vi "FeedbackDecode_MLComCtrl.vi"(6 "CognitiveLoadIn":T1, 8 "DecodeClustIn":T4={"TrainParams"={"Lag"=0.0, "KernelWidth"=0.3, "TargRad"=0.15}, "Kinematics"={"Thumb"=0.0, "Index"=0.0, "Middle"=0.0, "Ring"=0.0, "Little"=0.0, "ThumbInt"=0.0, "IndexInt"=0.0, "RingInt"=0.0, "LittleInt"=0.0, "Wrist"=0.0, "WristYaw"=0.0, "WristRoll"=0.0}, "CtrlButtons"={"AcqTraining"=FALSE, "ApplyBaseline"=FALSE, "ApplyTraining"=FALSE, "LoadTrainFile"=FALSE, "CAR"=FALSE, "NIPSpikes"=FALSE, "AcqBaseline"=FALSE, "Stop"=FALSE, "ResetTrial"=FALSE, "CalDEKA"=FALSE, "HideSphrs"=FALSE, "StartTrials"=FALSE, "AutoPop"=FALSE, "ResetVRE"=FALSE, "StopVRE"=FALSE, "AcqCAR"=FALSE, "ConARD"=FALSE, "DEKARestart"=FALSE, "ConnDEKA"=FALSE}, "CompID"={"LV"={"Name"="PNILABVIEW", "IP"="155.100.90.215"}, "ML"={"Name"="PNIMATLAB", "IP"="155.100.91.231"}}, "KMvntClust"={"KGain"=[[1.0, 1.0, -1.0, 1.0], [1.0, 1.0, -1.0, 1.0], [1.0, 1.0, -1.0, 1.0], [1.0, 1.0, -1.0, 1.0], [1.0, 1.0, -1.0, 1.0], [1.0, 1.0, -1.0, 1.0], [1.0, 1.0, -1.0, 1.0], [1.0, 1.0, -1.0, 1.0], [1.0, 1.0, -1.0, 1.0], [1.0, 1.0, -1.0, 1.0], [1.0, 1.0, -1.0, 1.0], [1.0, 1.0, -1.0, 1.0]], "KMvnts"={"Thumb"=FALSE, "Index"=FALSE, "Middle"=FALSE, "Ring"=FALSE, "Little"=FALSE, "ThumbInt"=FALSE, "IndexInt"=FALSE, "RingInt"=FALSE, "LittleInt"=FALSE, "WristPitch"=FALSE, "WristYaw"=FALSE, "WristRoll"=FALSE}, "KThresh"=[[0.2, 0.2, -1.0, 1.0], [0.2, 0.2, -1.0, 1.0], [0.2, 0.2, -1.0, 1.0], [0.2, 0.2, -1.0, 1.0], [0.2, 0.2, -1.0, 1.0], [0.2, 0.2, -1.0, 1.0], [0.2, 0.2, -1.0, 1.0], [0.2, 0.2, -1.0, 1.0], [0.2, 0.2, -1.0, 1.0], [0.2, 0.2, -1.0, 1.0], [0.2, 0.2, -1.0, 1.0], [0.2, 0.2, -1.0, 1.0]], "CtrlMode"=[], "CtrlSpd"=[]}, "ClearUEA"=FALSE, "Targets"={"Thumb"=0.0, "Index"=0.0, "Middle"=0.0, "Ring"=0.0, "Little"=0.0, "ThumbInt"=0.0, "IndexInt"=0.0, "RingInt"=0.0, "LittleInt"=0.0, "Wrist"=0.0, "WristYaw"=0.0, "WristRoll"=0.0}, "KUEAArray"=[{"Boolean 1"=FALSE, "Boolean 2"=FALSE, "Boolean 3"=FALSE, "Boolean 4"=FALSE, "Boolean 5"=FALSE, "Boolean 6"=FALSE, "Boolean 7"=FALSE, "Boolean 8"=FALSE, "Boolean 9"=FALSE, "Boolean 10"=FALSE, "Boolean 11"=FALSE, "Boolean 12"=FALSE, "Boolean 13"=FALSE, "Boolean 14"=FALSE, "Boolean 15"=FALSE, "Boolean 16"=FALSE, "Boolean 17"=FALSE, "Boolean 18"=FALSE, "Boolean 19"=FALSE, "Boolean 20"=FALSE, "Boolean 21"=FALSE, "Boolean 22"=FALSE, "Boolean 23"=FALSE, "Boolean 24"=FALSE, "Boolean 25"=FALSE, "Boolean 26"=FALSE, "Boolean 27"=FALSE, "Boolean 28"=FALSE, "Boolean 29"=FALSE, "Boolean 30"=FALSE, "Boolean 31"=FALSE, "Boolean 32"=FALSE, "Boolean 33"=FALSE, "Boolean 34"=FALSE, "Boolean 35"=FALSE, "Boolean 36"=FALSE, "Boolean 37"=FALSE, "Boolean 38"=FALSE, "Boolean 39"=FALSE, "Boolean 40"=FALSE, "Boolean 41"=FALSE, "Boolean 42"=FALSE, "Boolean 43"=FALSE, "Boolean 44"=FALSE, "Boolean 45"=FALSE, "Boolean 46"=FALSE, "Boolean 47"=FALSE, "Boolean 48"=FALSE, "Boolean 49"=FALSE, "Boolean 50"=FALSE, "Boolean 51"=FALSE, "Boolean 52"=FALSE, "Boolean 53"=FALSE, "Boolean 54"=FALSE, "Boolean 55"=FALSE, "Boolean 56"=FALSE, "Boolean 57"=FALSE, "Boolean 58"=FALSE, "Boolean 59"=FALSE, "Boolean 60"=FALSE, "Boolean 61"=FALSE, "Boolean 62"=FALSE, "Boolean 63"=FALSE, "Boolean 64"=FALSE, "Boolean 65"=FALSE, "Boolean 66"=FALSE, "Boolean 67"=FALSE, "Boolean 68"=FALSE, "Boolean 69"=FALSE, "Boolean 70"=FALSE, "Boolean 71"=FALSE, "Boolean 72"=FALSE, "Boolean 73"=FALSE, "Boolean 74"=FALSE, "Boolean 75"=FALSE, "Boolean 76"=FALSE, "Boolean 77"=FALSE, "Boolean 78"=FALSE, "Boolean 79"=FALSE, "Boolean 80"=FALSE, "Boolean 81"=FALSE, "Boolean 82"=FALSE, "Boolean 83"=FALSE, "Boolean 84"=FALSE, "Boolean 85"=FALSE, "Boolean 86"=FALSE, "Boolean 87"=FALSE, "Boolean 88"=FALSE, "Boolean 89"=FALSE, "Boolean 90"=FALSE, "Boolean 91"=FALSE, "Boolean 92"=FALSE, "Boolean 93"=FALSE, "Boolean 94"=FALSE, "Boolean 95"=FALSE, "Boolean 96"=FALSE, "Boolean 97"=FALSE, "Boolean 98"=FALSE, "Boolean 99"=FALSE, "Boolean 100"=FALSE}, {"Boolean 1"=FALSE, "Boolean 2"=FALSE, "Boolean 3"=FALSE, "Boolean 4"=FALSE, "Boolean 5"=FALSE, "Boolean 6"=FALSE, "Boolean 7"=FALSE, "Boolean 8"=FALSE, "Boolean 9"=FALSE, "Boolean 10"=FALSE, "Boolean 11"=FALSE, "Boolean 12"=FALSE, "Boolean 13"=FALSE, "Boolean 14"=FALSE, "Boolean 15"=FALSE, "Boolean 16"=FALSE, "Boolean 17"=FALSE, "Boolean 18"=FALSE, "Boolean 19"=FALSE, "Boolean 20"=FALSE, "Boolean 21"=FALSE, "Boolean 22"=FALSE, "Boolean 23"=FALSE, "Boolean 24"=FALSE, "Boolean 25"=FALSE, "Boolean 26"=FALSE, "Boolean 27"=FALSE, "Boolean 28"=FALSE, "Boolean 29"=FALSE, "Boolean 30"=FALSE, "Boolean 31"=FALSE, "Boolean 32"=FALSE, "Boolean 33"=FALSE, "Boolean 34"=FALSE, "Boolean 35"=FALSE, "Boolean 36"=FALSE, "Boolean 37"=FALSE, "Boolean 38"=FALSE, "Boolean 39"=FALSE, "Boolean 40"=FALSE, "Boolean 41"=FALSE, "Boolean 42"=FALSE, "Boolean 43"=FALSE, "Boolean 44"=FALSE, "Boolean 45"=FALSE, "Boolean 46"=FALSE, "Boolean 47"=FALSE, "Boolean 48"=FALSE, "Boolean 49"=FALSE, "Boolean 50"=FALSE, "Boolean 51"=FALSE, "Boolean 52"=FALSE, "Boolean 53"=FALSE, "Boolean 54"=FALSE, "Boolean 55"=FALSE, "Boolean 56"=FALSE, "Boolean 57"=FALSE, "Boolean 58"=FALSE, "Boolean 59"=FALSE, "Boolean 60"=FALSE, "Boolean 61"=FALSE, "Boolean 62"=FALSE, "Boolean 63"=FALSE, "Boolean 64"=FALSE, "Boolean 65"=FALSE, "Boolean 66"=FALSE, "Boolean 67"=FALSE, "Boolean 68"=FALSE, "Boolean 69"=FALSE, "Boolean 70"=FALSE, "Boolean 71"=FALSE, "Boolean 72"=FALSE, "Boolean 73"=FALSE, "Boolean 74"=FALSE, "Boolean 75"=FALSE, "Boolean 76"=FALSE, "Boolean 77"=FALSE, "Boolean 78"=FALSE, "Boolean 79"=FALSE, "Boolean 80"=FALSE, "Boolean 81"=FALSE, "Boolean 82"=FALSE, "Boolean 83"=FALSE, "Boolean 84"=FALSE, "Boolean 85"=FALSE, "Boolean 86"=FALSE, "Boolean 87"=FALSE, "Boolean 88"=FALSE, "Boolean 89"=FALSE, "Boolean 90"=FALSE, "Boolean 91"=FALSE, "Boolean 92"=FALSE, "Boolean 93"=FALSE, "Boolean 94"=FALSE, "Boolean 95"=FALSE, "Boolean 96"=FALSE, "Boolean 97"=FALSE, "Boolean 98"=FALSE, "Boolean 99"=FALSE, "Boolean 100"=FALSE}], "ReTrain"=FALSE, "TargDist"=[0.0, 0.0, 0.0, 0.0, 0.0, 0.0], "State"=enum."Initialize", "KalmanType"=enum."Standard", "EventStr"="", "SelElect"=1.0, "KinSrc"=enum."Training", "HoverElect"=0.0, "RasterWin"=1.0, "WfCnt"=15.0, "ClearWfs"=FALSE, "ApplyThresh"=FALSE, "ThreshVal"=-5.0, "ThreshMode"=enum."RMS Single", "DataFolder"="00000000-000000", "ClearEMG"=FALSE, "KEMGClust"={"Boolean 92"=FALSE, "Boolean 82"=FALSE, "Boolean 72"=FALSE, "Boolean 62"=FALSE, "Boolean 52"=FALSE, "Boolean 42"=FALSE, "Boolean 32"=FALSE, "Boolean 22"=FALSE, "Boolean 12"=FALSE, "Boolean 2"=FALSE, "Boolean 93"=FALSE, "Boolean 83"=FALSE, "Boolean 73"=FALSE, "Boolean 63"=FALSE, "Boolean 53"=FALSE, "Boolean 43"=FALSE, "Boolean 33"=FALSE, "Boolean 23"=FALSE, "Boolean 13"=FALSE, "Boolean 3"=FALSE, "Boolean 94"=FALSE, "Boolean 84"=FALSE, "Boolean 74"=FALSE, "Boolean 64"=FALSE, "Boolean 54"=FALSE, "Boolean 44"=FALSE, "Boolean 34"=FALSE, "Boolean 24"=FALSE, "Boolean 14"=FALSE, "Boolean 4"=FALSE, "Boolean 95"=FALSE, "Boolean 85"=FALSE, "Boolean 75"=FALSE, "Boolean 65"=FALSE, "Boolean 55"=FALSE, "Boolean 45"=FALSE, "Boolean 35"=FALSE, "Boolean 25"=FALSE, "Boolean 15"=FALSE, "Boolean 5"=FALSE, "Boolean 96"=FALSE, "Boolean 86"=FALSE, "Boolean 76"=FALSE, "Boolean 66"=FALSE, "Boolean 56"=FALSE, "Boolean 46"=FALSE, "Boolean 36"=FALSE, "Boolean 26"=FALSE, "Boolean 16"=FALSE, "Boolean 6"=FALSE, "Boolean 97"=FALSE, "Boolean 87"=FALSE, "Boolean 77"=FALSE, "Boolean 67"=FALSE, "Boolean 57"=FALSE, "Boolean 47"=FALSE, "Boolean 37"=FALSE, "Boolean 27"=FALSE, "Boolean 17"=FALSE, "Boolean 7"=FALSE, "Boolean 98"=FALSE, "Boolean 88"=FALSE, "Boolean 78"=FALSE, "Boolean 68"=FALSE, "Boolean 58"=FALSE, "Boolean 48"=FALSE, "Boolean 38"=FALSE, "Boolean 28"=FALSE, "Boolean 18"=FALSE, "Boolean 8"=FALSE, "Boolean 99"=FALSE, "Boolean 89"=FALSE, "Boolean 79"=FALSE, "Boolean 69"=FALSE, "Boolean 59"=FALSE, "Boolean 49"=FALSE, "Boolean 39"=FALSE, "Boolean 29"=FALSE, "Boolean 19"=FALSE, "Boolean 9"=FALSE}, "EvntFlag"=FALSE, "FillUEA"=FALSE, "FillEMG"=FALSE, "FillMvnts"=FALSE, "BadUEAElects"=[], "KEMGExtra"=[], "AllPairs"=FALSE, "AutoThresh"=0.4, "BadEMGChans"=[], "LinkedDOF"="{}", "AutoPopType"=enum."Standard", "CARType"=enum."Standard", "*Map"=enum."pNeural/pEMG", "GainFill"=1.0, "ThreshFill"=1.0, "TestType"=enum."MSMS", "Outcome"=enum."---", "TrialCnt"=[], "ClearTrials"=FALSE, "Log10"=FALSE, "KDFFile"="{}", "LimitExt"=FALSE, "*Prosthesis"=enum."MaleLeft", "StartML"=FALSE, "StartMLAux"=FALSE, "StartRec"=FALSE, "DynaThr"=FALSE, "ModeFill"=enum."Position", "SpdFill"=1.0, "DEKAMode"=enum."Velocity", "FreeParam"=0.4, "GoalNoise"=0.4, "Load NN"=FALSE, "ExportTrain"=FALSE, "NumComp"=enum."2 Computers", "DataDir"="00000000-000000", "BuildDir"="00000000-000000", "LatchingFilter"=FALSE, "Trigger"=FALSE, "StartARD"=FALSE, "StartTaska"=FALSE, "StartTaskaSens"=FALSE} {"SpdFill" min=0.0 max=10.0 step=0.1; "RasterWin" min=1.0 max=30.0 step=1.0; "ThreshFill" min=0.0 max=10.0 step=0.01; "GainFill" min=0.0 max=10.0 step=0.1; "AutoThresh" min=0.0 max=1.0; "Targets"."LittleInt" min=0.0 max=1.0 step=0.01; "Targets"."WristRoll" min=0.0 max=1.0 step=0.01; "Targets"."WristYaw" min=0.0 max=1.0 step=0.01; "Targets"."Wrist" min=0.0 max=1.0 step=0.01; "Targets"."Little" min=0.0 max=1.0 step=0.01; "Targets"."Thumb" min=0.0 max=1.0 step=0.01; "Targets"."RingInt" min=0.0 max=1.0 step=0.01; "Targets"."IndexInt" min=0.0 max=1.0 step=0.01; "Targets"."ThumbInt" min=0.0 max=1.0 step=0.01; "Targets"."Ring" min=0.0 max=1.0 step=0.01; "Targets"."Middle" min=0.0 max=1.0 step=0.01; "Targets"."Index" min=0.0 max=1.0 step=0.01; "KMvntClust"."CtrlSpd" min=0 max=10; "KMvntClust"."KThresh" min=0 max=1; "KMvntClust"."KGain" min=0; "Kinematics"."LittleInt" min=0.0 max=1.0 step=0.01; "Kinematics"."WristRoll" min=0.0 max=1.0 step=0.01; "Kinematics"."WristYaw" min=0.0 max=1.0 step=0.01; "Kinematics"."Wrist" min=0.0 max=1.0 step=0.01; "Kinematics"."Little" min=0.0 max=1.0 step=0.01; "Kinematics"."Thumb" min=0.0 max=1.0 step=0.01; "Kinematics"."RingInt" min=0.0 max=1.0 step=0.01; "Kinematics"."IndexInt" min=0.0 max=1.0 step=0.01; "Kinematics"."ThumbInt" min=0.0 max=1.0 step=0.01; "Kinematics"."Ring" min=0.0 max=1.0 step=0.01; "Kinematics"."Middle" min=0.0 max=1.0 step=0.01; "Kinematics"."Index" min=0.0 max=1.0 step=0.01; "TrainParams"."TargRad" step=0.05 format="%#.2g"; "TrainParams"."KernelWidth" step=0.05 format="%#.2g"}, 9 "EncodeClustIn":T3={"ParamsTable"=[], "Sel"=[], "Stim"=FALSE, "StimMode"=enum."Off", "StimStep"=[enum."1uA", enum."1uA", enum."Off"], "Jitter"=FALSE, "Pulse"=FALSE, "BFreq"=0.0, "BAmp"=0.0, "UEAArray"=[], "AdjClust"={"Add"=FALSE, "Sub"=FALSE, "Val"=[1.0, 100.0, 0.2, 500.0, 0.0], "B"=[FALSE, FALSE, FALSE, FALSE, FALSE], "Inc+"=["x+1", "x+10", "x+0.1", "x+10", "x+10"], "Set"=FALSE, "LoadTable"=FALSE, "SaveTable"=FALSE, "ClearTable"=FALSE, "DeleteSel"=FALSE, "Inc-"=["x-1", "x-10", "x-0.1", "x-10", "x-10"]}, "PresetTable"=[], "SelPreset"=[], "SortClust"={"Region"=FALSE, "Receptor"=FALSE, "Electrode"=FALSE, "Min Amp"=FALSE, "Max Amp"=FALSE, "Min Freq"=FALSE, "Max Freq"=FALSE, "Duration"=FALSE}, "SelSort"={"Sel"=FALSE}, "PresetClust"={"Load"=FALSE, "Clear"=FALSE, "Save"=FALSE, "Del"=FALSE}, "RespClust"={"RespType"=enum."Sensor Map", "OpenResp"=FALSE}, "AmpLimit"=0.0, "FreqLimit"=0.0, "DurLimit"=0.0, "Wait Period"=0.0, "Train Period"=0.0, "ManualType"=enum."Max"} {"Train Period" min=0.0 max=100.0 step=0.1; "Wait Period" min=0.0 max=100.0 step=0.1; "DurLimit" min=0.0 max=1.0 step=0.01; "FreqLimit" min=0.0 max=500.0 step=1.0; "AmpLimit" min=0.0 max=100.0 step=1.0; "BAmp" min=0.0 max=100.0 step=1.0; "BFreq" min=0.0 max=100.0 step=1.0}, 10 "ManualDOF":T2, 11 "Mode":T6(ring)=enum."SendEvent") -> (0 "DecodeClustOut":T4={"TrainParams"={"Lag"=0.0, "KernelWidth"=0.3, "TargRad"=0.15}, "Kinematics"={"Thumb"=0.0, "Index"=0.0, "Middle"=0.0, "Ring"=0.0, "Little"=0.0, "ThumbInt"=0.0, "IndexInt"=0.0, "RingInt"=0.0, "LittleInt"=0.0, "Wrist"=0.0, "WristYaw"=0.0, "WristRoll"=0.0}, "CtrlButtons"={"AcqTraining"=FALSE, "ApplyBaseline"=FALSE, "ApplyTraining"=FALSE, "LoadTrainFile"=FALSE, "CAR"=FALSE, "NIPSpikes"=FALSE, "AcqBaseline"=FALSE, "Stop"=FALSE, "ResetTrial"=FALSE, "CalDEKA"=FALSE, "HideSphrs"=FALSE, "StartTrials"=FALSE, "AutoPop"=FALSE, "ResetVRE"=FALSE, "StopVRE"=FALSE, "AcqCAR"=FALSE, "ConARD"=FALSE, "DEKARestart"=FALSE, "ConnDEKA"=FALSE}, "CompID"={"LV"={"Name"="PNILABVIEW", "IP"="155.100.90.215"}, "ML"={"Name"="PNIMATLAB", "IP"="155.100.91.231"}}, "KMvntClust"={"KGain"=[[1.0, 1.0, -1.0, 1.0], [1.0, 1.0, -1.0, 1.0], [1.0, 1.0, -1.0, 1.0], [1.0, 1.0, -1.0, 1.0], [1.0, 1.0, -1.0, 1.0], [1.0, 1.0, -1.0, 1.0], [1.0, 1.0, -1.0, 1.0], [1.0, 1.0, -1.0, 1.0], [1.0, 1.0, -1.0, 1.0], [1.0, 1.0, -1.0, 1.0], [1.0, 1.0, -1.0, 1.0], [1.0, 1.0, -1.0, 1.0]], "KMvnts"={"Thumb"=FALSE, "Index"=FALSE, "Middle"=FALSE, "Ring"=FALSE, "Little"=FALSE, "ThumbInt"=FALSE, "IndexInt"=FALSE, "RingInt"=FALSE, "LittleInt"=FALSE, "WristPitch"=FALSE, "WristYaw"=FALSE, "WristRoll"=FALSE}, "KThresh"=[[0.2, 0.2, -1.0, 1.0], [0.2, 0.2, -1.0, 1.0], [0.2, 0.2, -1.0, 1.0], [0.2, 0.2, -1.0, 1.0], [0.2, 0.2, -1.0, 1.0], [0.2, 0.2, -1.0, 1.0], [0.2, 0.2, -1.0, 1.0], [0.2, 0.2, -1.0, 1.0], [0.2, 0.2, -1.0, 1.0], [0.2, 0.2, -1.0, 1.0], [0.2, 0.2, -1.0, 1.0], [0.2, 0.2, -1.0, 1.0]], "CtrlMode"=[], "CtrlSpd"=[]}, "ClearUEA"=FALSE, "Targets"={"Thumb"=0.0, "Index"=0.0, "Middle"=0.0, "Ring"=0.0, "Little"=0.0, "ThumbInt"=0.0, "IndexInt"=0.0, "RingInt"=0.0, "LittleInt"=0.0, "Wrist"=0.0, "WristYaw"=0.0, "WristRoll"=0.0}, "KUEAArray"=[{"Boolean 1"=FALSE, "Boolean 2"=FALSE, "Boolean 3"=FALSE, "Boolean 4"=FALSE, "Boolean 5"=FALSE, "Boolean 6"=FALSE, "Boolean 7"=FALSE, "Boolean 8"=FALSE, "Boolean 9"=FALSE, "Boolean 10"=FALSE, "Boolean 11"=FALSE, "Boolean 12"=FALSE, "Boolean 13"=FALSE, "Boolean 14"=FALSE, "Boolean 15"=FALSE, "Boolean 16"=FALSE, "Boolean 17"=FALSE, "Boolean 18"=FALSE, "Boolean 19"=FALSE, "Boolean 20"=FALSE, "Boolean 21"=FALSE, "Boolean 22"=FALSE, "Boolean 23"=FALSE, "Boolean 24"=FALSE, "Boolean 25"=FALSE, "Boolean 26"=FALSE, "Boolean 27"=FALSE, "Boolean 28"=FALSE, "Boolean 29"=FALSE, "Boolean 30"=FALSE, "Boolean 31"=FALSE, "Boolean 32"=FALSE, "Boolean 33"=FALSE, "Boolean 34"=FALSE, "Boolean 35"=FALSE, "Boolean 36"=FALSE, "Boolean 37"=FALSE, "Boolean 38"=FALSE, "Boolean 39"=FALSE, "Boolean 40"=FALSE, "Boolean 41"=FALSE, "Boolean 42"=FALSE, "Boolean 43"=FALSE, "Boolean 44"=FALSE, "Boolean 45"=FALSE, "Boolean 46"=FALSE, "Boolean 47"=FALSE, "Boolean 48"=FALSE, "Boolean 49"=FALSE, "Boolean 50"=FALSE, "Boolean 51"=FALSE, "Boolean 52"=FALSE, "Boolean 53"=FALSE, "Boolean 54"=FALSE, "Boolean 55"=FALSE, "Boolean 56"=FALSE, "Boolean 57"=FALSE, "Boolean 58"=FALSE, "Boolean 59"=FALSE, "Boolean 60"=FALSE, "Boolean 61"=FALSE, "Boolean 62"=FALSE, "Boolean 63"=FALSE, "Boolean 64"=FALSE, "Boolean 65"=FALSE, "Boolean 66"=FALSE, "Boolean 67"=FALSE, "Boolean 68"=FALSE, "Boolean 69"=FALSE, "Boolean 70"=FALSE, "Boolean 71"=FALSE, "Boolean 72"=FALSE, "Boolean 73"=FALSE, "Boolean 74"=FALSE, "Boolean 75"=FALSE, "Boolean 76"=FALSE, "Boolean 77"=FALSE, "Boolean 78"=FALSE, "Boolean 79"=FALSE, "Boolean 80"=FALSE, "Boolean 81"=FALSE, "Boolean 82"=FALSE, "Boolean 83"=FALSE, "Boolean 84"=FALSE, "Boolean 85"=FALSE, "Boolean 86"=FALSE, "Boolean 87"=FALSE, "Boolean 88"=FALSE, "Boolean 89"=FALSE, "Boolean 90"=FALSE, "Boolean 91"=FALSE, "Boolean 92"=FALSE, "Boolean 93"=FALSE, "Boolean 94"=FALSE, "Boolean 95"=FALSE, "Boolean 96"=FALSE, "Boolean 97"=FALSE, "Boolean 98"=FALSE, "Boolean 99"=FALSE, "Boolean 100"=FALSE}, {"Boolean 1"=FALSE, "Boolean 2"=FALSE, "Boolean 3"=FALSE, "Boolean 4"=FALSE, "Boolean 5"=FALSE, "Boolean 6"=FALSE, "Boolean 7"=FALSE, "Boolean 8"=FALSE, "Boolean 9"=FALSE, "Boolean 10"=FALSE, "Boolean 11"=FALSE, "Boolean 12"=FALSE, "Boolean 13"=FALSE, "Boolean 14"=FALSE, "Boolean 15"=FALSE, "Boolean 16"=FALSE, "Boolean 17"=FALSE, "Boolean 18"=FALSE, "Boolean 19"=FALSE, "Boolean 20"=FALSE, "Boolean 21"=FALSE, "Boolean 22"=FALSE, "Boolean 23"=FALSE, "Boolean 24"=FALSE, "Boolean 25"=FALSE, "Boolean 26"=FALSE, "Boolean 27"=FALSE, "Boolean 28"=FALSE, "Boolean 29"=FALSE, "Boolean 30"=FALSE, "Boolean 31"=FALSE, "Boolean 32"=FALSE, "Boolean 33"=FALSE, "Boolean 34"=FALSE, "Boolean 35"=FALSE, "Boolean 36"=FALSE, "Boolean 37"=FALSE, "Boolean 38"=FALSE, "Boolean 39"=FALSE, "Boolean 40"=FALSE, "Boolean 41"=FALSE, "Boolean 42"=FALSE, "Boolean 43"=FALSE, "Boolean 44"=FALSE, "Boolean 45"=FALSE, "Boolean 46"=FALSE, "Boolean 47"=FALSE, "Boolean 48"=FALSE, "Boolean 49"=FALSE, "Boolean 50"=FALSE, "Boolean 51"=FALSE, "Boolean 52"=FALSE, "Boolean 53"=FALSE, "Boolean 54"=FALSE, "Boolean 55"=FALSE, "Boolean 56"=FALSE, "Boolean 57"=FALSE, "Boolean 58"=FALSE, "Boolean 59"=FALSE, "Boolean 60"=FALSE, "Boolean 61"=FALSE, "Boolean 62"=FALSE, "Boolean 63"=FALSE, "Boolean 64"=FALSE, "Boolean 65"=FALSE, "Boolean 66"=FALSE, "Boolean 67"=FALSE, "Boolean 68"=FALSE, "Boolean 69"=FALSE, "Boolean 70"=FALSE, "Boolean 71"=FALSE, "Boolean 72"=FALSE, "Boolean 73"=FALSE, "Boolean 74"=FALSE, "Boolean 75"=FALSE, "Boolean 76"=FALSE, "Boolean 77"=FALSE, "Boolean 78"=FALSE, "Boolean 79"=FALSE, "Boolean 80"=FALSE, "Boolean 81"=FALSE, "Boolean 82"=FALSE, "Boolean 83"=FALSE, "Boolean 84"=FALSE, "Boolean 85"=FALSE, "Boolean 86"=FALSE, "Boolean 87"=FALSE, "Boolean 88"=FALSE, "Boolean 89"=FALSE, "Boolean 90"=FALSE, "Boolean 91"=FALSE, "Boolean 92"=FALSE, "Boolean 93"=FALSE, "Boolean 94"=FALSE, "Boolean 95"=FALSE, "Boolean 96"=FALSE, "Boolean 97"=FALSE, "Boolean 98"=FALSE, "Boolean 99"=FALSE, "Boolean 100"=FALSE}], "ReTrain"=FALSE, "TargDist"=[0.0, 0.0, 0.0, 0.0, 0.0, 0.0], "State"=enum."Initialize", "KalmanType"=enum."Standard", "EventStr"="", "SelElect"=1.0, "KinSrc"=enum."Training", "HoverElect"=0.0, "RasterWin"=1.0, "WfCnt"=15.0, "ClearWfs"=FALSE, "ApplyThresh"=FALSE, "ThreshVal"=-5.0, "ThreshMode"=enum."RMS Single", "DataFolder"="00000000-000000", "ClearEMG"=FALSE, "KEMGClust"={"Boolean 92"=FALSE, "Boolean 82"=FALSE, "Boolean 72"=FALSE, "Boolean 62"=FALSE, "Boolean 52"=FALSE, "Boolean 42"=FALSE, "Boolean 32"=FALSE, "Boolean 22"=FALSE, "Boolean 12"=FALSE, "Boolean 2"=FALSE, "Boolean 93"=FALSE, "Boolean 83"=FALSE, "Boolean 73"=FALSE, "Boolean 63"=FALSE, "Boolean 53"=FALSE, "Boolean 43"=FALSE, "Boolean 33"=FALSE, "Boolean 23"=FALSE, "Boolean 13"=FALSE, "Boolean 3"=FALSE, "Boolean 94"=FALSE, "Boolean 84"=FALSE, "Boolean 74"=FALSE, "Boolean 64"=FALSE, "Boolean 54"=FALSE, "Boolean 44"=FALSE, "Boolean 34"=FALSE, "Boolean 24"=FALSE, "Boolean 14"=FALSE, "Boolean 4"=FALSE, "Boolean 95"=FALSE, "Boolean 85"=FALSE, "Boolean 75"=FALSE, "Boolean 65"=FALSE, "Boolean 55"=FALSE, "Boolean 45"=FALSE, "Boolean 35"=FALSE, "Boolean 25"=FALSE, "Boolean 15"=FALSE, "Boolean 5"=FALSE, "Boolean 96"=FALSE, "Boolean 86"=FALSE, "Boolean 76"=FALSE, "Boolean 66"=FALSE, "Boolean 56"=FALSE, "Boolean 46"=FALSE, "Boolean 36"=FALSE, "Boolean 26"=FALSE, "Boolean 16"=FALSE, "Boolean 6"=FALSE, "Boolean 97"=FALSE, "Boolean 87"=FALSE, "Boolean 77"=FALSE, "Boolean 67"=FALSE, "Boolean 57"=FALSE, "Boolean 47"=FALSE, "Boolean 37"=FALSE, "Boolean 27"=FALSE, "Boolean 17"=FALSE, "Boolean 7"=FALSE, "Boolean 98"=FALSE, "Boolean 88"=FALSE, "Boolean 78"=FALSE, "Boolean 68"=FALSE, "Boolean 58"=FALSE, "Boolean 48"=FALSE, "Boolean 38"=FALSE, "Boolean 28"=FALSE, "Boolean 18"=FALSE, "Boolean 8"=FALSE, "Boolean 99"=FALSE, "Boolean 89"=FALSE, "Boolean 79"=FALSE, "Boolean 69"=FALSE, "Boolean 59"=FALSE, "Boolean 49"=FALSE, "Boolean 39"=FALSE, "Boolean 29"=FALSE, "Boolean 19"=FALSE, "Boolean 9"=FALSE}, "EvntFlag"=FALSE, "FillUEA"=FALSE, "FillEMG"=FALSE, "FillMvnts"=FALSE, "BadUEAElects"=[], "KEMGExtra"=[], "AllPairs"=FALSE, "AutoThresh"=0.4, "BadEMGChans"=[], "LinkedDOF"="{}", "AutoPopType"=enum."Standard", "CARType"=enum."Standard", "*Map"=enum."pNeural/pEMG", "GainFill"=1.0, "ThreshFill"=1.0, "TestType"=enum."MSMS", "Outcome"=enum."---", "TrialCnt"=[], "ClearTrials"=FALSE, "Log10"=FALSE, "KDFFile"="{}", "LimitExt"=FALSE, "*Prosthesis"=enum."MaleLeft", "StartML"=FALSE, "StartMLAux"=FALSE, "StartRec"=FALSE, "DynaThr"=FALSE, "ModeFill"=enum."Position", "SpdFill"=1.0, "DEKAMode"=enum."Velocity", "FreeParam"=0.4, "GoalNoise"=0.4, "Load NN"=FALSE, "ExportTrain"=FALSE, "NumComp"=enum."2 Computers", "DataDir"="00000000-000000", "BuildDir"="00000000-000000", "LatchingFilter"=FALSE, "Trigger"=FALSE, "StartARD"=FALSE, "StartTaska"=FALSE, "StartTaskaSens"=FALSE} {"SpdFill" min=0.0 max=10.0 step=0.1; "RasterWin" min=1.0 max=30.0 step=1.0; "ThreshFill" min=0.0 max=10.0 step=0.01; "GainFill" min=0.0 max=10.0 step=0.1; "AutoThresh" min=0.0 max=1.0; "Targets"."LittleInt" min=0.0 max=1.0 step=0.01; "Targets"."WristRoll" min=0.0 max=1.0 step=0.01; "Targets"."WristYaw" min=0.0 max=1.0 step=0.01; "Targets"."Wrist" min=0.0 max=1.0 step=0.01; "Targets"."Little" min=0.0 max=1.0 step=0.01; "Targets"."Thumb" min=0.0 max=1.0 step=0.01; "Targets"."RingInt" min=0.0 max=1.0 step=0.01; "Targets"."IndexInt" min=0.0 max=1.0 step=0.01; "Targets"."ThumbInt" min=0.0 max=1.0 step=0.01; "Targets"."Ring" min=0.0 max=1.0 step=0.01; "Targets"."Middle" min=0.0 max=1.0 step=0.01; "Targets"."Index" min=0.0 max=1.0 step=0.01; "KMvntClust"."CtrlSpd" min=0 max=10; "KMvntClust"."KThresh" min=0 max=1; "KMvntClust"."KGain" min=0; "Kinematics"."LittleInt" min=0.0 max=1.0 step=0.01; "Kinematics"."WristRoll" min=0.0 max=1.0 step=0.01; "Kinematics"."WristYaw" min=0.0 max=1.0 step=0.01; "Kinematics"."Wrist" min=0.0 max=1.0 step=0.01; "Kinematics"."Little" min=0.0 max=1.0 step=0.01; "Kinematics"."Thumb" min=0.0 max=1.0 step=0.01; "Kinematics"."RingInt" min=0.0 max=1.0 step=0.01; "Kinematics"."IndexInt" min=0.0 max=1.0 step=0.01; "Kinematics"."ThumbInt" min=0.0 max=1.0 step=0.01; "Kinematics"."Ring" min=0.0 max=1.0 step=0.01; "Kinematics"."Middle" min=0.0 max=1.0 step=0.01; "Kinematics"."Index" min=0.0 max=1.0 step=0.01; "TrainParams"."TargRad" step=0.05 format="%#.2g"; "TrainParams"."KernelWidth" step=0.05 format="%#.2g"}, 1 "EncodeClustOut":T3={"ParamsTable"=[], "Sel"=[], "Stim"=FALSE, "StimMode"=enum."Off", "StimStep"=[enum."1uA", enum."1uA", enum."Off"], "Jitter"=FALSE, "Pulse"=FALSE, "BFreq"=0.0, "BAmp"=0.0, "UEAArray"=[], "AdjClust"={"Add"=FALSE, "Sub"=FALSE, "Val"=[1.0, 100.0, 0.2, 500.0, 0.0], "B"=[FALSE, FALSE, FALSE, FALSE, FALSE], "Inc+"=["x+1", "x+10", "x+0.1", "x+10", "x+10"], "Set"=FALSE, "LoadTable"=FALSE, "SaveTable"=FALSE, "ClearTable"=FALSE, "DeleteSel"=FALSE, "Inc-"=["x-1", "x-10", "x-0.1", "x-10", "x-10"]}, "PresetTable"=[], "SelPreset"=[], "SortClust"={"Region"=FALSE, "Receptor"=FALSE, "Electrode"=FALSE, "Min Amp"=FALSE, "Max Amp"=FALSE, "Min Freq"=FALSE, "Max Freq"=FALSE, "Duration"=FALSE}, "SelSort"={"Sel"=FALSE}, "PresetClust"={"Load"=FALSE, "Clear"=FALSE, "Save"=FALSE, "Del"=FALSE}, "RespClust"={"RespType"=enum."Sensor Map", "OpenResp"=FALSE}, "AmpLimit"=0.0, "FreqLimit"=0.0, "DurLimit"=0.0, "Wait Period"=0.0, "Train Period"=0.0, "ManualType"=enum."Max"} {"Train Period" min=0.0 max=100.0 step=0.1; "Wait Period" min=0.0 max=100.0 step=0.1; "DurLimit" min=0.0 max=1.0 step=0.01; "FreqLimit" min=0.0 max=500.0 step=1.0; "AmpLimit" min=0.0 max=100.0 step=1.0; "BAmp" min=0.0 max=100.0 step=1.0; "BFreq" min=0.0 max=100.0 step=1.0}, 3 "MLClust":T5={"LoopTimings"={"MLCalcTime"=0.0, "MLTotalTime"=0.3}, "Kalman"={"Thumb"=0.0, "Index"=0.0, "Middle"=0.0, "Ring"=0.0, "Little"=0.0, "ThumbInt"=0.0, "IndexInt"=0.0, "RingInt"=0.0, "LittleInt"=0.0, "Wrist"=0.0, "WristYaw"=0.0, "WristRoll"=0.0}, "Kinematics"={"Thumb"=0.0, "Index"=0.0, "Middle"=0.0, "Ring"=0.0, "Little"=0.0, "ThumbInt"=0.0, "IndexInt"=0.0, "RingInt"=0.0, "LittleInt"=0.0, "Wrist"=0.0, "WristYaw"=0.0, "WristRoll"=0.0}, "ElectRates"=[], "SelWfs"=[], "TrainCnt"=0.3, "EMGPwr"=[], "SelData"=[], "SelRate"=[], "SelKin"=[], "NIPTime"=0.3, "VREID"=0, "StimWf"=[], "RawDecodeOutput"=[], "TASKA IR sensors"=[], "TASKA baro sensors"=[]} {"VREID" step=1; "NIPTime" step=0.05 format="%#.2g"; "TrainCnt" step=0.05 format="%#.2g"; "Kinematics"."LittleInt" min=0.0 max=1.0 step=0.01; "Kinematics"."WristRoll" min=0.0 max=1.0 step=0.01; "Kinematics"."WristYaw" min=0.0 max=1.0 step=0.01; "Kinematics"."Wrist" min=0.0 max=1.0 step=0.01; "Kinematics"."Little" min=0.0 max=1.0 step=0.01; "Kinematics"."Thumb" min=0.0 max=1.0 step=0.01; "Kinematics"."RingInt" min=0.0 max=1.0 step=0.01; "Kinematics"."IndexInt" min=0.0 max=1.0 step=0.01; "Kinematics"."ThumbInt" min=0.0 max=1.0 step=0.01; "Kinematics"."Ring" min=0.0 max=1.0 step=0.01; "Kinematics"."Middle" min=0.0 max=1.0 step=0.01; "Kinematics"."Index" min=0.0 max=1.0 step=0.01; "Kalman"."LittleInt" min=0.0 max=1.0 step=0.01; "Kalman"."WristRoll" min=0.0 max=1.0 step=0.01; "Kalman"."WristYaw" min=0.0 max=1.0 step=0.01; "Kalman"."Wrist" min=0.0 max=1.0 step=0.01; "Kalman"."Little" min=0.0 max=1.0 step=0.01; "Kalman"."Thumb" min=0.0 max=1.0 step=0.01; "Kalman"."RingInt" min=0.0 max=1.0 step=0.01; "Kalman"."IndexInt" min=0.0 max=1.0 step=0.01; "Kalman"."ThumbInt" min=0.0 max=1.0 step=0.01; "Kalman"."Ring" min=0.0 max=1.0 step=0.01; "Kalman"."Middle" min=0.0 max=1.0 step=0.01; "Kalman"."Index" min=0.0 max=1.0 step=0.01; "LoopTimings"."MLTotalTime" step=0.05 format="%#.2g"}, 4 "CognitiveLoadOut":T1)   [LabVIEW 2020]
uses:
  FeedbackDecode_DecodeClust.ctl
  FeedbackDecode_EncodeClust.ctl
  FeedbackDecode_CogLoadClust.ctl
  FeedbackDecode_VariablesToString_Scalar.vi
  FeedbackDecode_VariablesToString_String.vi
  FeedbackDecode_VariablesToString_Array.vi
  FeedbackDecode_Globals.vi
panel:
  out "UDPCont":refnum<k16>
  out "ML.IP":string
  out "LV.IP":string
  out "UDPEvnt":refnum<k16>
  # "Note: Pupillometry glasses must be connected prior to starting FeedbackDecode"
  # "Note: Pupillometry glasses must be connected prior to starting FeedbackDecode"
  # "Value"
  # "Inc-"
  # "Inc+"
  # "Min Amp"
  # "Max Amp"
  # "Min Freq"
  # "Max Freq"
  # "Duration"
  # "Value"
  # "Inc-"
  # "Inc+"
  # "Min Amp"
  # "Max Amp"
  # "Min Freq"
  # "Max Freq"
  # "Duration"
  # "G"
  # "T"
  # "Mode"
  # "S"
  # "Negative lag shifts feature variables left (earlier)"
  # "{[1,2,4];[5,3];[6,7,8]}"
  # "Select before apply training"
  # "1"
  # "2"
  # "3"
  # "4"
  # "5"
  # "6"
  # "7"
  # "8"
  # "1"
  # "2"
  # "3"
  # "4"
  # "1-2"
  # "1-3"
  # "1-4"
  # "2-3"
  # "2-4"
  # "3-4"
  # "DOF"
  # "Gain (F/E)"
  # "Thresh (F/E)"
  # "Mode"
  # "Spd"
  # "G"
  # "T"
  # "Mode"
  # "S"
  # "Negative lag shifts feature variables left (earlier)"
  # "{[1,2,4];[5,3];[6,7,8]}"
  # "Select before apply training"
  # "1"
  # "2"
  # "3"
  # "4"
  # "5"
  # "6"
  # "7"
  # "8"
  # "1"
  # "2"
  # "3"
  # "4"
  # "1-2"
  # "1-3"
  # "1-4"
  # "2-3"
  # "2-4"
  # "3-4"
  # "DOF"
  # "Gain (F/E)"
  # "Thresh (F/E)"
  # "Mode"
  # "Spd"
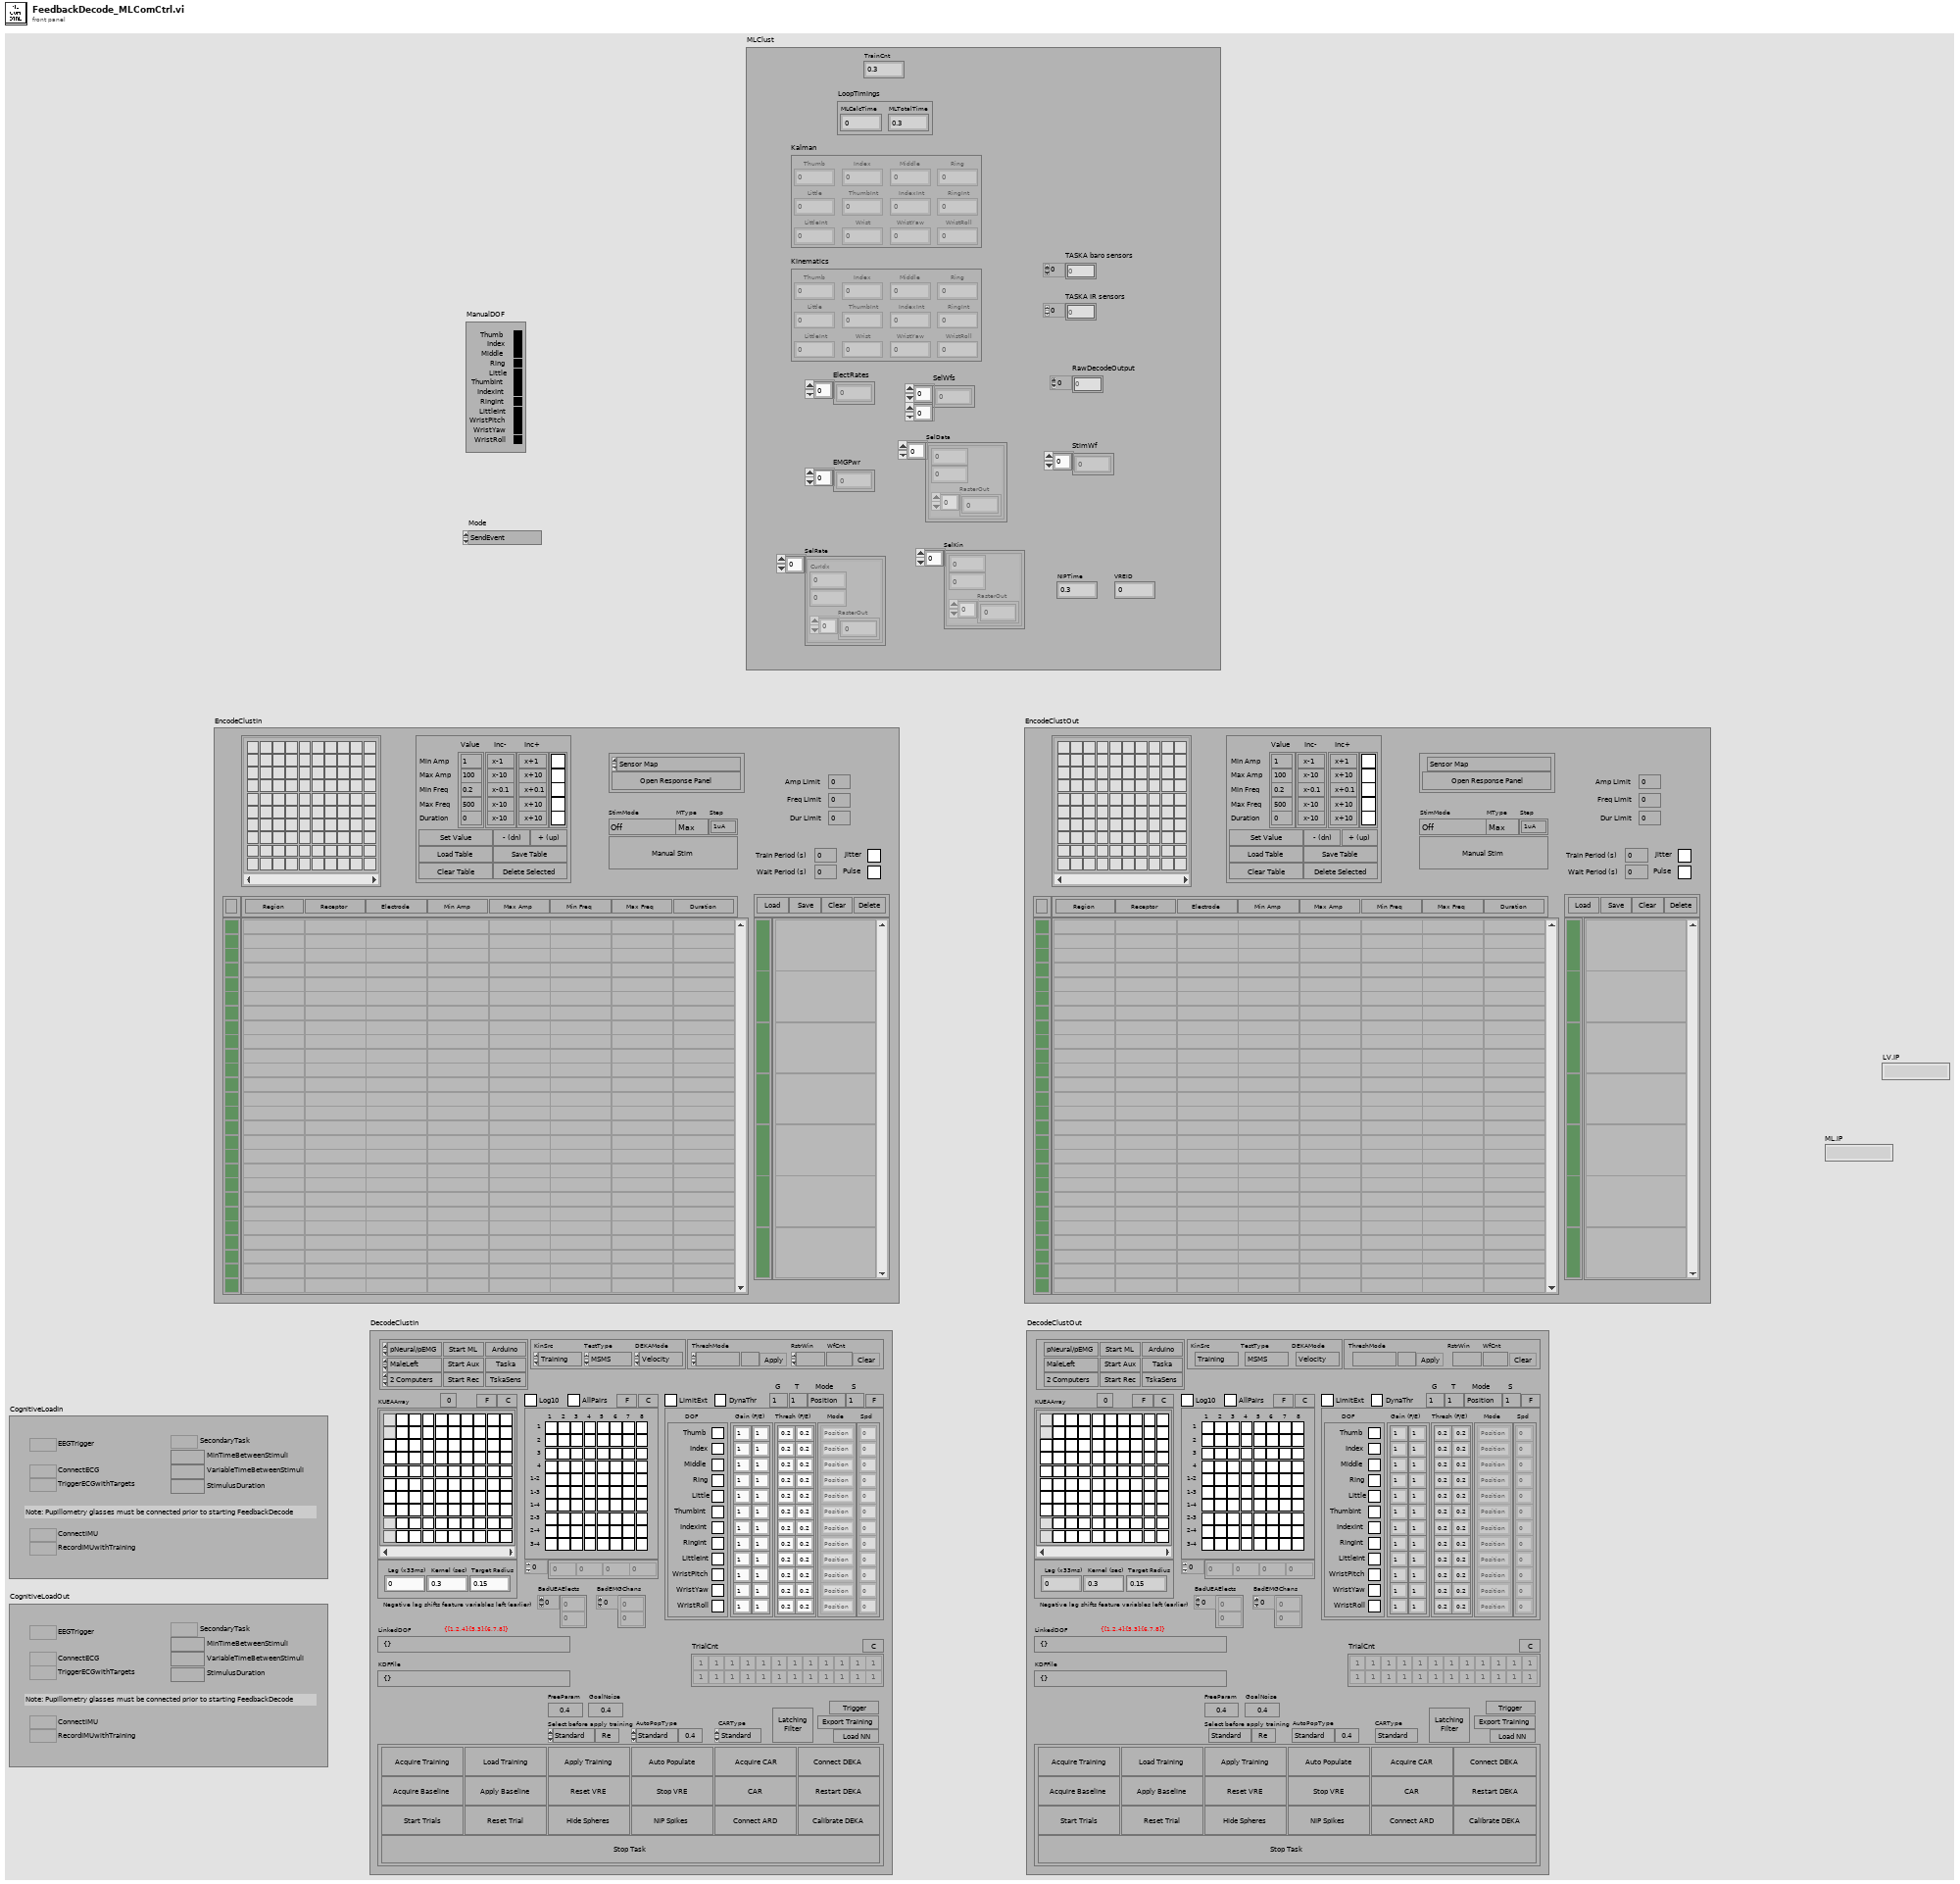
[diagram p1: front panel]
types:
  T1 = typedef "FeedbackDecode_CogLoadClust.ctl" = cluster{"EEGTrigger":bool, "ConnectECG":bool, "TriggerECGwithTargets":bool, "SecondaryTask":bool, "MinTimeBetweenStimuli":dbl, "VariableTimeBetweenStimuli":dbl, "StimulusDuration":dbl, "RecordIMUwithTraining":bool, "ConnectIMU":bool}
  T2 = cluster{"Thumb":enum8{"False", "True", "Mixed"}, "Index":enum8{"False", "True", "Mixed"}, "Middle":enum8{"False", "True", "Mixed"}, "Ring":enum8{"False", "True", "Mixed"}, "Little":enum8{"False", "True", "Mixed"}, "ThumbInt":enum8{"False", "True", "Mixed"}, "IndexInt":enum8{"False", "True", "Mixed"}, "RingInt":enum8{"False", "True", "Mixed"}, "LittleInt":enum8{"False", "True", "Mixed"}, "WristPitch":enum8{"False", "True", "Mixed"}, "WristYaw":enum8{"False", "True", "Mixed"}, "WristRoll":enum8{"False", "True", "Mixed"}}
  T3 = typedef "FeedbackDecode_EncodeClust.ctl" = cluster{"ParamsTable":string[][], "Sel":bool[], "Stim":bool, "StimMode":enum16{"Off", "Manual", "MSMS", "VRE", "3DHand", "DEKA", "Analog(DEKA)"}, "StimStep":enum16{"Off", "1uA", "2uA", "5uA", "10uA", "20uA", "30uA"}[], "Jitter":bool, "Pulse":bool, "BFreq":dbl, "BAmp":dbl, "UEAArray":cluster{"Boolean 1":bool, "Boolean 2":bool, "Boolean 3":bool, "Boolean 4":bool, "Boolean 5":bool, "Boolean 6":bool, "Boolean 7":bool, "Boolean 8":bool, "Boolean 9":bool, "Boolean 10":bool, "Boolean 11":bool, "Boolean 12":bool, "Boolean 13":bool, "Boolean 14":bool, "Boolean 15":bool, "Boolean 16":bool, "Boolean 17":bool, "Boolean 18":bool, "Boolean 19":bool, "Boolean 20":bool, "Boolean 21":bool, "Boolean 22":bool, "Boolean 23":bool, "Boolean 24":bool, "Boolean 25":bool, "Boolean 26":bool, "Boolean 27":bool, "Boolean 28":bool, "Boolean 29":bool, "Boolean 30":bool, "Boolean 31":bool, "Boolean 32":bool, "Boolean 33":bool, "Boolean 34":bool, "Boolean 35":bool, "Boolean 36":bool, "Boolean 37":bool, "Boolean 38":bool, "Boolean 39":bool, "Boolean 40":bool, "Boolean 41":bool, "Boolean 42":bool, "Boolean 43":bool, "Boolean 44":bool, "Boolean 45":bool, "Boolean 46":bool, "Boolean 47":bool, "Boolean 48":bool, "Boolean 49":bool, "Boolean 50":bool, "Boolean 51":bool, "Boolean 52":bool, "Boolean 53":bool, "Boolean 54":bool, "Boolean 55":bool, "Boolean 56":bool, "Boolean 57":bool, "Boolean 58":bool, "Boolean 59":bool, "Boolean 60":bool, "Boolean 61":bool, "Boolean 62":bool, "Boolean 63":bool, "Boolean 64":bool, "Boolean 65":bool, "Boolean 66":bool, "Boolean 67":bool, "Boolean 68":bool, "Boolean 69":bool, "Boolean 70":bool, "Boolean 71":bool, "Boolean 72":bool, "Boolean 73":bool, "Boolean 74":bool, "Boolean 75":bool, "Boolean 76":bool, "Boolean 77":bool, "Boolean 78":bool, "Boolean 79":bool, "Boolean 80":bool, "Boolean 81":bool, "Boolean 82":bool, "Boolean 83":bool, "Boolean 84":bool, "Boolean 85":bool, "Boolean 86":bool, "Boolean 87":bool, "Boolean 88":bool, "Boolean 89":bool, "Boolean 90":bool, "Boolean 91":bool, "Boolean 92":bool, "Boolean 93":bool, "Boolean 94":bool, "Boolean 95":bool, "Boolean 96":bool, "Boolean 97":bool, "Boolean 98":bool, "Boolean 99":bool, "Boolean 100":bool}[], "AdjClust":cluster{"Add":bool, "Sub":bool, "Val":dbl[], "B":bool[], "Inc+":string[], "Set":bool, "LoadTable":bool, "SaveTable":bool, "ClearTable":bool, "DeleteSel":bool, "Inc-":string[]}, "PresetTable":string[][], "SelPreset":bool[], "SortClust":cluster{"Region":bool, "Receptor":bool, "Electrode":bool, "Min Amp":bool, "Max Amp":bool, "Min Freq":bool, "Max Freq":bool, "Duration":bool}, "SelSort":cluster{"Sel":bool}, "PresetClust":cluster{"Load":bool, "Clear":bool, "Save":bool, "Del":bool}, "RespClust":cluster{"RespType":enum16{"Sensor Map", "Full Map"}, "OpenResp":bool}, "AmpLimit":dbl, "FreqLimit":dbl, "DurLimit":dbl, "Wait Period":dbl, "Train Period":dbl, "ManualType":enum16{"Max", "Min"}}
  T4 = typedef "FeedbackDecode_DecodeClust.ctl" = cluster{"TrainParams":cluster{"Lag":dbl, "KernelWidth":dbl, "TargRad":dbl}, "Kinematics":cluster{"Thumb":dbl, "Index":dbl, "Middle":dbl, "Ring":dbl, "Little":dbl, "ThumbInt":dbl, "IndexInt":dbl, "RingInt":dbl, "LittleInt":dbl, "Wrist":dbl, "WristYaw":dbl, "WristRoll":dbl}, "CtrlButtons":cluster{"AcqTraining":bool, "ApplyBaseline":bool, "ApplyTraining":bool, "LoadTrainFile":bool, "CAR":bool, "NIPSpikes":bool, "AcqBaseline":bool, "Stop":bool, "ResetTrial":bool, "CalDEKA":bool, "HideSphrs":bool, "StartTrials":bool, "AutoPop":bool, "ResetVRE":bool, "StopVRE":bool, "AcqCAR":bool, "ConARD":bool, "DEKARestart":bool, "ConnDEKA":bool}, "CompID":cluster{"LV":cluster{"Name":string, "IP":string}, "ML":cluster{"Name":string, "IP":string}}, "KMvntClust":cluster{"KGain":sgl[][], "KMvnts":cluster{"Thumb":bool, "Index":bool, "Middle":bool, "Ring":bool, "Little":bool, "ThumbInt":bool, "IndexInt":bool, "RingInt":bool, "LittleInt":bool, "WristPitch":bool, "WristYaw":bool, "WristRoll":bool}, "KThresh":sgl[][], "CtrlMode":enum16{"Position", "Latching", "Leaky", "Velocity"}[], "CtrlSpd":sgl[]}, "ClearUEA":bool, "Targets":cluster{"Thumb":dbl, "Index":dbl, "Middle":dbl, "Ring":dbl, "Little":dbl, "ThumbInt":dbl, "IndexInt":dbl, "RingInt":dbl, "LittleInt":dbl, "Wrist":dbl, "WristYaw":dbl, "WristRoll":dbl}, "KUEAArray":cluster{"Boolean 1":bool, "Boolean 2":bool, "Boolean 3":bool, "Boolean 4":bool, "Boolean 5":bool, "Boolean 6":bool, "Boolean 7":bool, "Boolean 8":bool, "Boolean 9":bool, "Boolean 10":bool, "Boolean 11":bool, "Boolean 12":bool, "Boolean 13":bool, "Boolean 14":bool, "Boolean 15":bool, "Boolean 16":bool, "Boolean 17":bool, "Boolean 18":bool, "Boolean 19":bool, "Boolean 20":bool, "Boolean 21":bool, "Boolean 22":bool, "Boolean 23":bool, "Boolean 24":bool, "Boolean 25":bool, "Boolean 26":bool, "Boolean 27":bool, "Boolean 28":bool, "Boolean 29":bool, "Boolean 30":bool, "Boolean 31":bool, "Boolean 32":bool, "Boolean 33":bool, "Boolean 34":bool, "Boolean 35":bool, "Boolean 36":bool, "Boolean 37":bool, "Boolean 38":bool, "Boolean 39":bool, "Boolean 40":bool, "Boolean 41":bool, "Boolean 42":bool, "Boolean 43":bool, "Boolean 44":bool, "Boolean 45":bool, "Boolean 46":bool, "Boolean 47":bool, "Boolean 48":bool, "Boolean 49":bool, "Boolean 50":bool, "Boolean 51":bool, "Boolean 52":bool, "Boolean 53":bool, "Boolean 54":bool, "Boolean 55":bool, "Boolean 56":bool, "Boolean 57":bool, "Boolean 58":bool, "Boolean 59":bool, "Boolean 60":bool, "Boolean 61":bool, "Boolean 62":bool, "Boolean 63":bool, "Boolean 64":bool, "Boolean 65":bool, "Boolean 66":bool, "Boolean 67":bool, "Boolean 68":bool, "Boolean 69":bool, "Boolean 70":bool, "Boolean 71":bool, "Boolean 72":bool, "Boolean 73":bool, "Boolean 74":bool, "Boolean 75":bool, "Boolean 76":bool, "Boolean 77":bool, "Boolean 78":bool, "Boolean 79":bool, "Boolean 80":bool, "Boolean 81":bool, "Boolean 82":bool, "Boolean 83":bool, "Boolean 84":bool, "Boolean 85":bool, "Boolean 86":bool, "Boolean 87":bool, "Boolean 88":bool, "Boolean 89":bool, "Boolean 90":bool, "Boolean 91":bool, "Boolean 92":bool, "Boolean 93":bool, "Boolean 94":bool, "Boolean 95":bool, "Boolean 96":bool, "Boolean 97":bool, "Boolean 98":bool, "Boolean 99":bool, "Boolean 100":bool}[], "ReTrain":bool, "TargDist":dbl[], "State":enum16{"Initialize", "Acquire Start", "Acquire Response", "Finalize"}, "KalmanType":enum16{"Standard", "Mean", "Refit", "LinSVReg", "NonLinSVReg", "PCA", "DWPRR", "AdaptKF", "NN", "NN_python", "AdaptKF2", "KF_Short_Goal"}, "EventStr":string, "SelElect":dbl, "KinSrc":enum16{"Off", "Training", "Decode", "COB", "LEAP"}, "HoverElect":dbl, "RasterWin":dbl, "WfCnt":dbl, "ClearWfs":bool, "ApplyThresh":bool, "ThreshVal":dbl, "ThreshMode":enum16{"RMS Single", "RMS All", "RMS Auto", "Volt Single", "Volt All"}, "DataFolder":string, "ClearEMG":bool, "KEMGClust":cluster{"Boolean 92":bool, "Boolean 82":bool, "Boolean 72":bool, "Boolean 62":bool, "Boolean 52":bool, "Boolean 42":bool, "Boolean 32":bool, "Boolean 22":bool, "Boolean 12":bool, "Boolean 2":bool, "Boolean 93":bool, "Boolean 83":bool, "Boolean 73":bool, "Boolean 63":bool, "Boolean 53":bool, "Boolean 43":bool, "Boolean 33":bool, "Boolean 23":bool, "Boolean 13":bool, "Boolean 3":bool, "Boolean 94":bool, "Boolean 84":bool, "Boolean 74":bool, "Boolean 64":bool, "Boolean 54":bool, "Boolean 44":bool, "Boolean 34":bool, "Boolean 24":bool, "Boolean 14":bool, "Boolean 4":bool, "Boolean 95":bool, "Boolean 85":bool, "Boolean 75":bool, "Boolean 65":bool, "Boolean 55":bool, "Boolean 45":bool, "Boolean 35":bool, "Boolean 25":bool, "Boolean 15":bool, "Boolean 5":bool, "Boolean 96":bool, "Boolean 86":bool, "Boolean 76":bool, "Boolean 66":bool, "Boolean 56":bool, "Boolean 46":bool, "Boolean 36":bool, "Boolean 26":bool, "Boolean 16":bool, "Boolean 6":bool, "Boolean 97":bool, "Boolean 87":bool, "Boolean 77":bool, "Boolean 67":bool, "Boolean 57":bool, "Boolean 47":bool, "Boolean 37":bool, "Boolean 27":bool, "Boolean 17":bool, "Boolean 7":bool, "Boolean 98":bool, "Boolean 88":bool, "Boolean 78":bool, "Boolean 68":bool, "Boolean 58":bool, "Boolean 48":bool, "Boolean 38":bool, "Boolean 28":bool, "Boolean 18":bool, "Boolean 8":bool, "Boolean 99":bool, "Boolean 89":bool, "Boolean 79":bool, "Boolean 69":bool, "Boolean 59":bool, "Boolean 49":bool, "Boolean 39":bool, "Boolean 29":bool, "Boolean 19":bool, "Boolean 9":bool}, "EvntFlag":bool, "FillUEA":bool, "FillEMG":bool, "FillMvnts":bool, "BadUEAElects":dbl[], "KEMGExtra":dbl[], "AllPairs":bool, "AutoThresh":dbl, "BadEMGChans":dbl[], "LinkedDOF":string, "AutoPopType":enum16{"Standard", "Stepwise", "Gram"}, "CARType":enum16{"Standard", "NN"}, "*Map":enum16{"pNeural/pEMG", "pNeural/aEMG", "aNeural/pEMG", "aNeural/aEMG", "N2021/pEMG"}, "GainFill":dbl, "ThreshFill":dbl, "TestType":enum16{"MSMS", "Bakeoff11", "Bakeoff21", "Bakeoff31", "Bakeoff32", "Bakeoff32_Ball", "Bakeoff32_Checkers", "Bakeoff32_Pen", "FragileBlock"}, "Outcome":enum16{"---", "Success", "Failure"}, "TrialCnt":dbl[][], "ClearTrials":bool, "Log10":bool, "KDFFile":string, "LimitExt":bool, "*Prosthesis":enum16{"MaleRight", "MaleLeft"}, "StartML":bool, "StartMLAux":bool, "StartRec":bool, "DynaThr":bool, "ModeFill":enum16{"Position", "Latching", "Leaky", "Velocity"}, "SpdFill":dbl, "DEKAMode":enum16{"Velocity", "Position"}, "FreeParam":dbl, "GoalNoise":dbl, "Load NN":bool, "ExportTrain":bool, "NumComp":enum16{"1 Computer", "2 Computers"}, "DataDir":string, "BuildDir":string, "LatchingFilter":bool, "Trigger":bool, "StartARD":bool, "StartTaska":bool, "StartTaskaSens":bool}
  T5 = cluster{"LoopTimings":cluster{"MLCalcTime":dbl, "MLTotalTime":dbl}, "Kalman":cluster{"Thumb":dbl, "Index":dbl, "Middle":dbl, "Ring":dbl, "Little":dbl, "ThumbInt":dbl, "IndexInt":dbl, "RingInt":dbl, "LittleInt":dbl, "Wrist":dbl, "WristYaw":dbl, "WristRoll":dbl}, "Kinematics":cluster{"Thumb":dbl, "Index":dbl, "Middle":dbl, "Ring":dbl, "Little":dbl, "ThumbInt":dbl, "IndexInt":dbl, "RingInt":dbl, "LittleInt":dbl, "Wrist":dbl, "WristYaw":dbl, "WristRoll":dbl}, "ElectRates":dbl[], "SelWfs":dbl[][], "TrainCnt":dbl, "EMGPwr":dbl[], "SelData":cluster{dbl, dbl, "RasterOut":dbl[]}[], "SelRate":cluster{"CurIdx":dbl, dbl, "RasterOut":dbl[]}[], "SelKin":cluster{dbl, dbl, "RasterOut":dbl[]}[], "NIPTime":dbl, "VREID":i16, "StimWf":dbl[], "RawDecodeOutput":dbl[], "TASKA IR sensors":dbl[], "TASKA baro sensors":dbl[]}
  T6 = enum16{"Initialize", "Wait", "BuildInitStr", "BuildKalmanStr", "BuildStimStr", "BuildEMGStr", "GetEvent", "SendEvent", "ContIO", "LoadTrainFile", "CopyTraining", "Close"}
  T7 = cluster{"AcqTraining":bool, "ApplyBaseline":bool, "ApplyTraining":bool, "LoadTrainFile":bool, "CAR":bool, "NIPSpikes":bool, "AcqBaseline":bool, "Stop":bool, "ResetTrial":bool, "TrialSphrs":bool, "HideSphrs":bool, "StartTrials":bool, "AutoPop":bool, "ResetVRE":bool, "StopVRE":bool, "AcqCAR":bool, "ConARD":bool, "Empty2":bool, "Empty1":bool}
  T8 = cluster{"Boolean 1":bool, "Boolean 2":bool, "Boolean 3":bool, "Boolean 4":bool, "Boolean 5":bool, "Boolean 6":bool, "Boolean 7":bool, "Boolean 8":bool, "Boolean 9":bool, "Boolean 10":bool, "Boolean 11":bool, "Boolean 12":bool, "Boolean 13":bool, "Boolean 14":bool, "Boolean 15":bool, "Boolean 16":bool, "Boolean 17":bool, "Boolean 18":bool, "Boolean 19":bool, "Boolean 20":bool, "Boolean 21":bool, "Boolean 22":bool, "Boolean 23":bool, "Boolean 24":bool, "Boolean 25":bool, "Boolean 26":bool, "Boolean 27":bool, "Boolean 28":bool, "Boolean 29":bool, "Boolean 30":bool, "Boolean 31":bool, "Boolean 32":bool, "Boolean 33":bool, "Boolean 34":bool, "Boolean 35":bool, "Boolean 36":bool, "Boolean 37":bool, "Boolean 38":bool, "Boolean 39":bool, "Boolean 40":bool, "Boolean 41":bool, "Boolean 42":bool, "Boolean 43":bool, "Boolean 44":bool, "Boolean 45":bool, "Boolean 46":bool, "Boolean 47":bool, "Boolean 48":bool, "Boolean 49":bool, "Boolean 50":bool, "Boolean 51":bool, "Boolean 52":bool, "Boolean 53":bool, "Boolean 54":bool, "Boolean 55":bool, "Boolean 56":bool, "Boolean 57":bool, "Boolean 58":bool, "Boolean 59":bool, "Boolean 60":bool, "Boolean 61":bool, "Boolean 62":bool, "Boolean 63":bool, "Boolean 64":bool, "Boolean 65":bool, "Boolean 66":bool, "Boolean 67":bool, "Boolean 68":bool, "Boolean 69":bool, "Boolean 70":bool, "Boolean 71":bool, "Boolean 72":bool, "Boolean 73":bool, "Boolean 74":bool, "Boolean 75":bool, "Boolean 76":bool, "Boolean 77":bool, "Boolean 78":bool, "Boolean 79":bool, "Boolean 80":bool, "Boolean 81":bool, "Boolean 82":bool, "Boolean 83":bool, "Boolean 84":bool, "Boolean 85":bool, "Boolean 86":bool, "Boolean 87":bool, "Boolean 88":bool, "Boolean 89":bool, "Boolean 90":bool, "Boolean 91":bool, "Boolean 92":bool, "Boolean 93":bool, "Boolean 94":bool, "Boolean 95":bool, "Boolean 96":bool, "Boolean 97":bool, "Boolean 98":bool, "Boolean 99":bool, "Boolean 100":bool}[]
  T9 = cluster{"KGain":sgl[][], "KMvnts":cluster{"Thumb":bool, "Index":bool, "Middle":bool, "Ring":bool, "Little":bool, "ThumbInt":bool, "IndexInt":bool, "RingInt":bool, "LittleInt":bool, "WristPitch":bool, "WristYaw":bool, "WristRoll":bool}, "KThresh":sgl[][], "CtrlMode":enum16{"Position", "Latching", "Leaky", "Velocity"}[], "CtrlSpd":sgl[]}
  T10 = cluster{"Lag":dbl, "KernelWidth":dbl, "TargRad":dbl}
  T11 = enum16{"RMS Single", "RMS All", "RMS Auto", "Volt Single", "Volt All"}
  T12 = cluster{"AcqTraining":bool, "ApplyBaseline":bool, "ApplyTraining":bool, "LoadTrainFile":bool, "CAR":bool, "NIPSpikes":bool, "AcqBaseline":bool, "Stop":bool, "ResetTrial":bool, "CalDEKA":bool, "HideSphrs":bool, "StartTrials":bool, "AutoPop":bool, "ResetVRE":bool, "StopVRE":bool, "AcqCAR":bool, "ConARD":bool, "DEKARestart":bool, "ConnDEKA":bool}
  T13 = enum16{"Standard", "Mean", "Refit", "LinSVReg", "NonLinSVReg", "PCA", "DWPRR", "AdaptKF", "NN", "NN_python", "AdaptKF2", "KF_Short_Goal"}
  T14 = cluster{"Boolean 92":bool, "Boolean 82":bool, "Boolean 72":bool, "Boolean 62":bool, "Boolean 52":bool, "Boolean 42":bool, "Boolean 32":bool, "Boolean 22":bool, "Boolean 12":bool, "Boolean 2":bool, "Boolean 93":bool, "Boolean 83":bool, "Boolean 73":bool, "Boolean 63":bool, "Boolean 53":bool, "Boolean 43":bool, "Boolean 33":bool, "Boolean 23":bool, "Boolean 13":bool, "Boolean 3":bool, "Boolean 94":bool, "Boolean 84":bool, "Boolean 74":bool, "Boolean 64":bool, "Boolean 54":bool, "Boolean 44":bool, "Boolean 34":bool, "Boolean 24":bool, "Boolean 14":bool, "Boolean 4":bool, "Boolean 95":bool, "Boolean 85":bool, "Boolean 75":bool, "Boolean 65":bool, "Boolean 55":bool, "Boolean 45":bool, "Boolean 35":bool, "Boolean 25":bool, "Boolean 15":bool, "Boolean 5":bool, "Boolean 96":bool, "Boolean 86":bool, "Boolean 76":bool, "Boolean 66":bool, "Boolean 56":bool, "Boolean 46":bool, "Boolean 36":bool, "Boolean 26":bool, "Boolean 16":bool, "Boolean 6":bool, "Boolean 97":bool, "Boolean 87":bool, "Boolean 77":bool, "Boolean 67":bool, "Boolean 57":bool, "Boolean 47":bool, "Boolean 37":bool, "Boolean 27":bool, "Boolean 17":bool, "Boolean 7":bool, "Boolean 98":bool, "Boolean 88":bool, "Boolean 78":bool, "Boolean 68":bool, "Boolean 58":bool, "Boolean 48":bool, "Boolean 38":bool, "Boolean 28":bool, "Boolean 18":bool, "Boolean 8":bool, "Boolean 99":bool, "Boolean 89":bool, "Boolean 79":bool, "Boolean 69":bool, "Boolean 59":bool, "Boolean 49":bool, "Boolean 39":bool, "Boolean 29":bool, "Boolean 19":bool, "Boolean 9":bool}
  T15 = enum16{"Off", "Training", "Decode", "COB", "LEAP"}
  T16 = enum16{"pNeural/pEMG", "pNeural/aEMG", "aNeural/pEMG", "aNeural/aEMG", "N2021/pEMG"}
  T17 = enum16{"MSMS", "Bakeoff11", "Bakeoff21", "Bakeoff31", "Bakeoff32", "Bakeoff32_Ball", "Bakeoff32_Checkers", "Bakeoff32_Pen", "FragileBlock"}
  T18 = cluster{"Thumb":dbl, "Index":dbl, "Middle":dbl, "Ring":dbl, "Little":dbl, "ThumbInt":dbl, "IndexInt":dbl, "RingInt":dbl, "LittleInt":dbl, "Wrist":dbl, "WristYaw":dbl, "WristRoll":dbl}
  T19 = cluster{"[0]":sgl, "[1]":sgl, "[2]":sgl, "[3]":sgl, "[4]":sgl, "[5]":sgl, "[6]":sgl, "[7]":sgl, "[8]":sgl, "[9]":sgl, "[10]":sgl, "[11]":sgl}
  T20 = cluster{"Position":cluster{"WriRot":dbl, "WriPitch":dbl, "IndFlex":dbl, "MRPFlex":dbl, "ThuRawPitch":dbl, "ThuRawYaw":dbl, "ThuYaw":dbl, "ThuPitch":dbl}, "Force":cluster{"IndLat":dbl, "IndTip":dbl, "MidTip":dbl, "RinTip":dbl, "PinkyTip":dbl, "PalmDist":dbl, "PalmProx":dbl, "HandEdge":dbl, "HandDorsal":dbl, "ThuUlnar":dbl, "ThuRadial":dbl, "ThuTip":dbl, "ThuDorsal":dbl}}
  T21 = enum16{"Initialize", "Acquire Start", "Acquire Response", "Finalize"}
  T22 = cluster{"IndLat":dbl, "IndTip":dbl, "MidTip":dbl, "RinTip":dbl, "PinkyTip":dbl, "PalmDist":dbl, "PalmProx":dbl, "HandEdge":dbl, "HandDorsal":dbl, "ThuUlnar":dbl, "ThuRadial":dbl, "ThuTip":dbl, "ThuDorsal":dbl}
  T23 = cluster{"WriRot":dbl, "WriPitch":dbl, "IndFlex":dbl, "MRPFlex":dbl, "ThuRawPitch":dbl, "ThuRawYaw":dbl, "ThuYaw":dbl, "ThuPitch":dbl}
  T24 = cluster{"CurIdx":dbl, "RasterWin":dbl, "RasterOut":dbl[]}[]
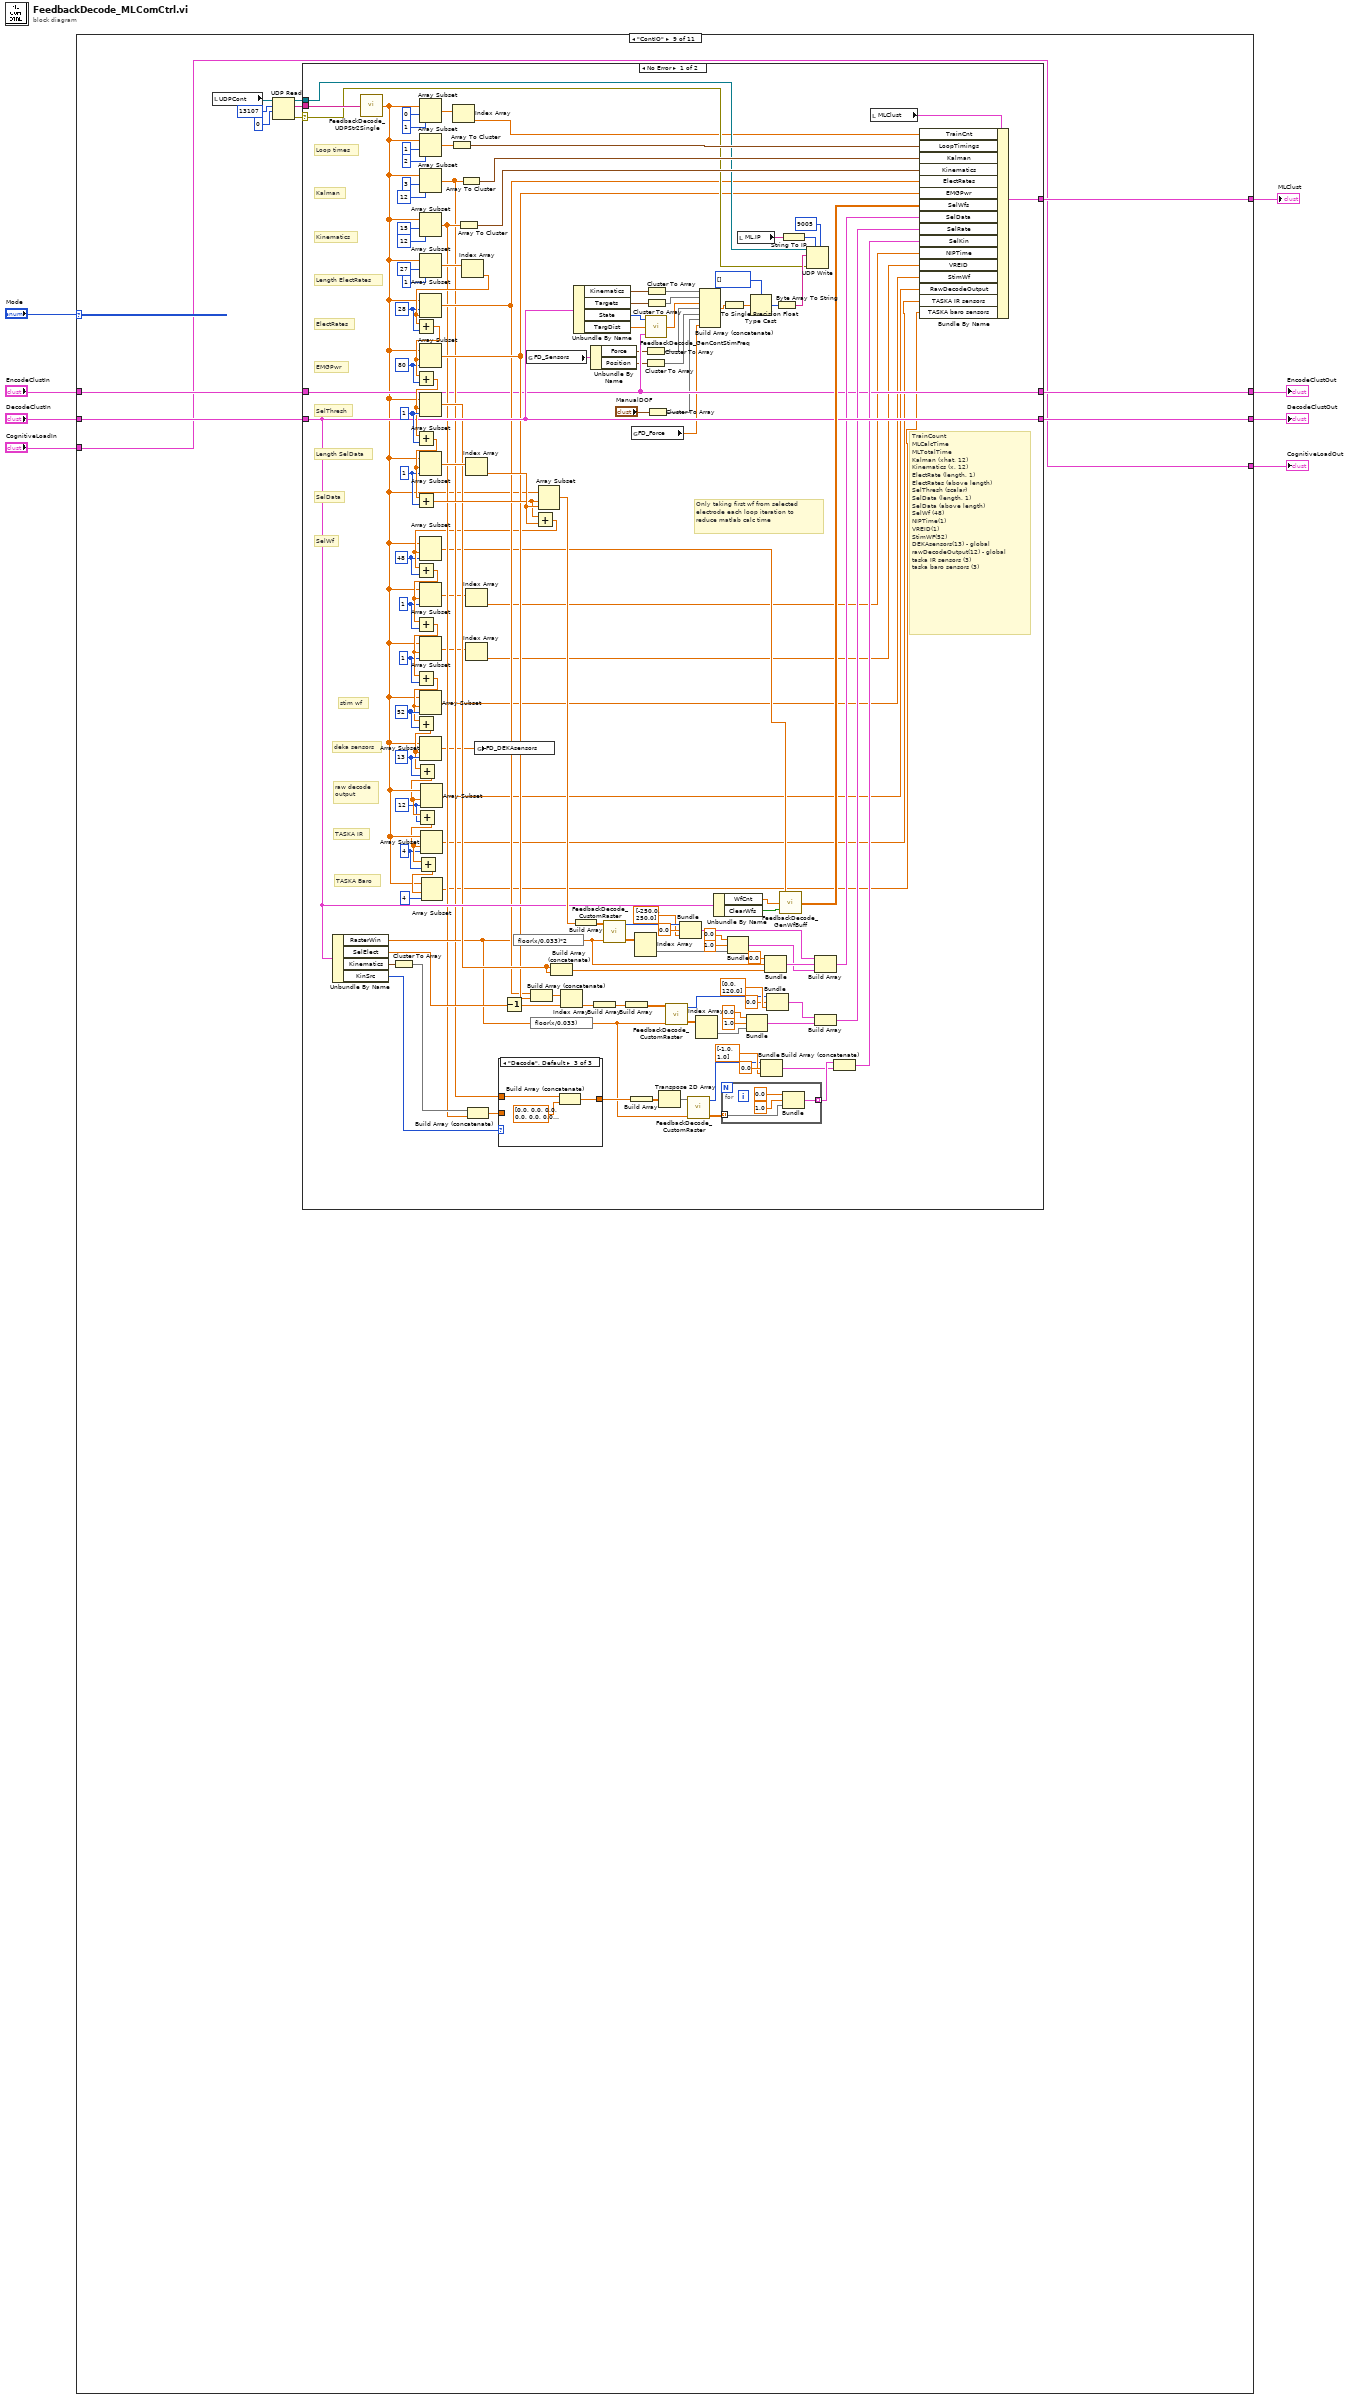
[diagram p0: block diagram]
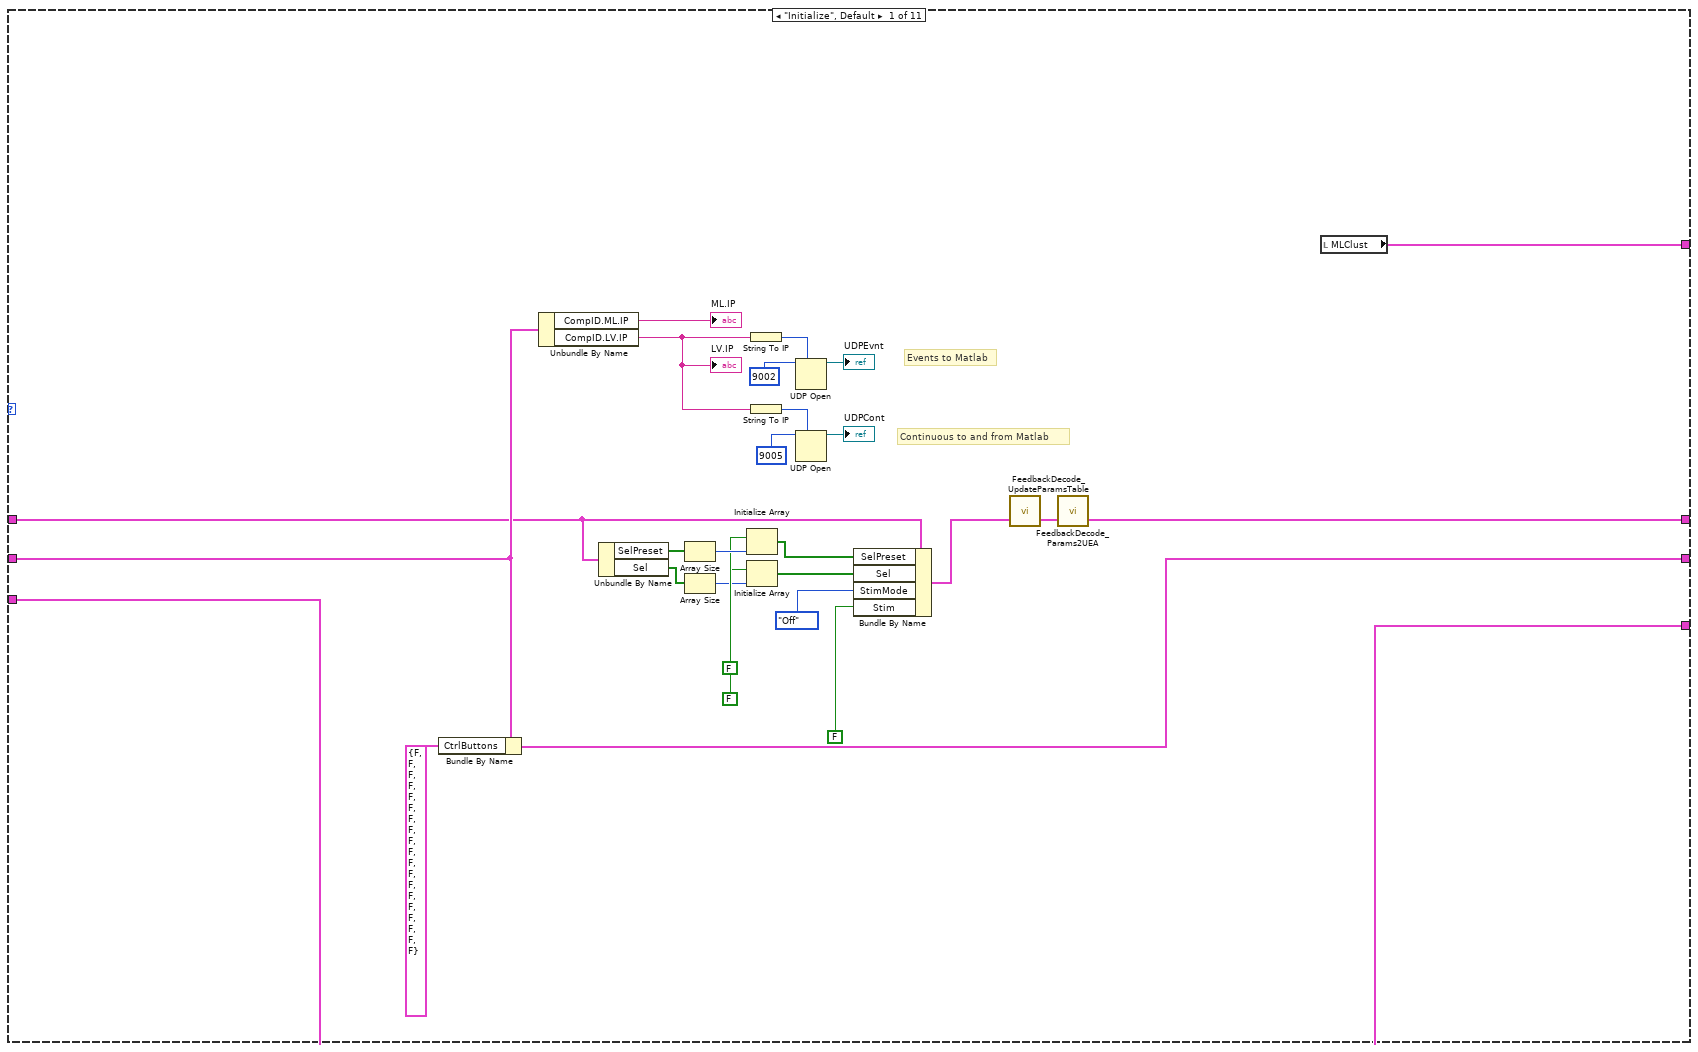
[diagram p2: hidden frame]
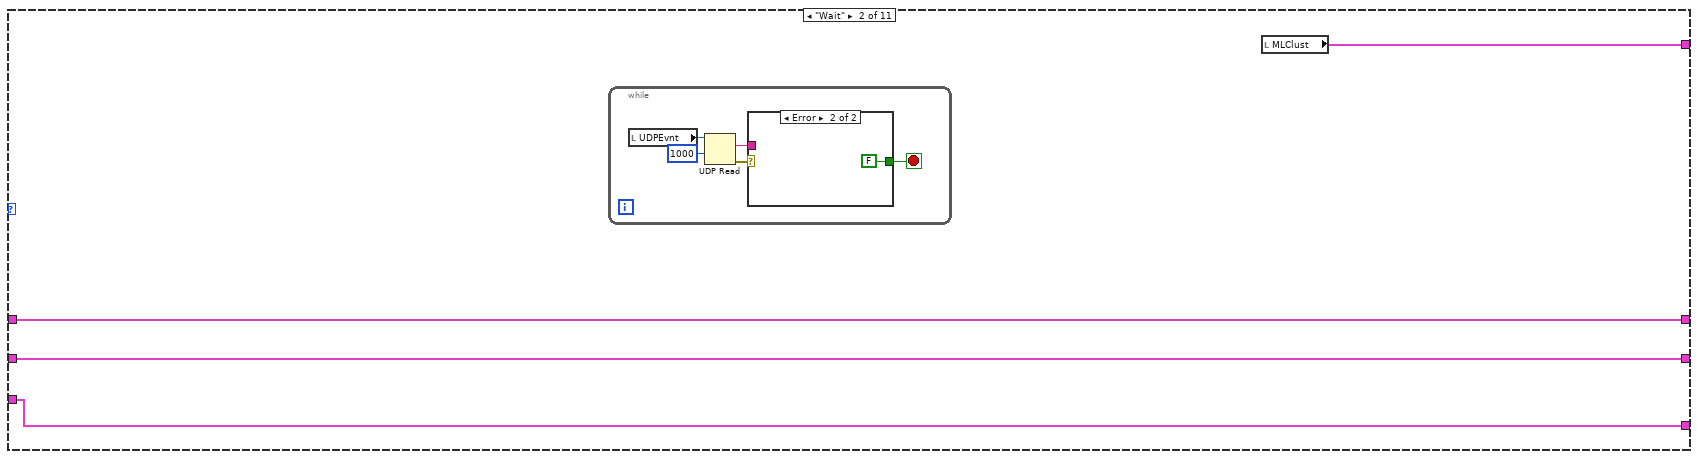
[diagram p3: hidden frame]
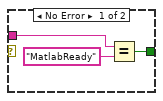
[diagram p4: hidden frame]
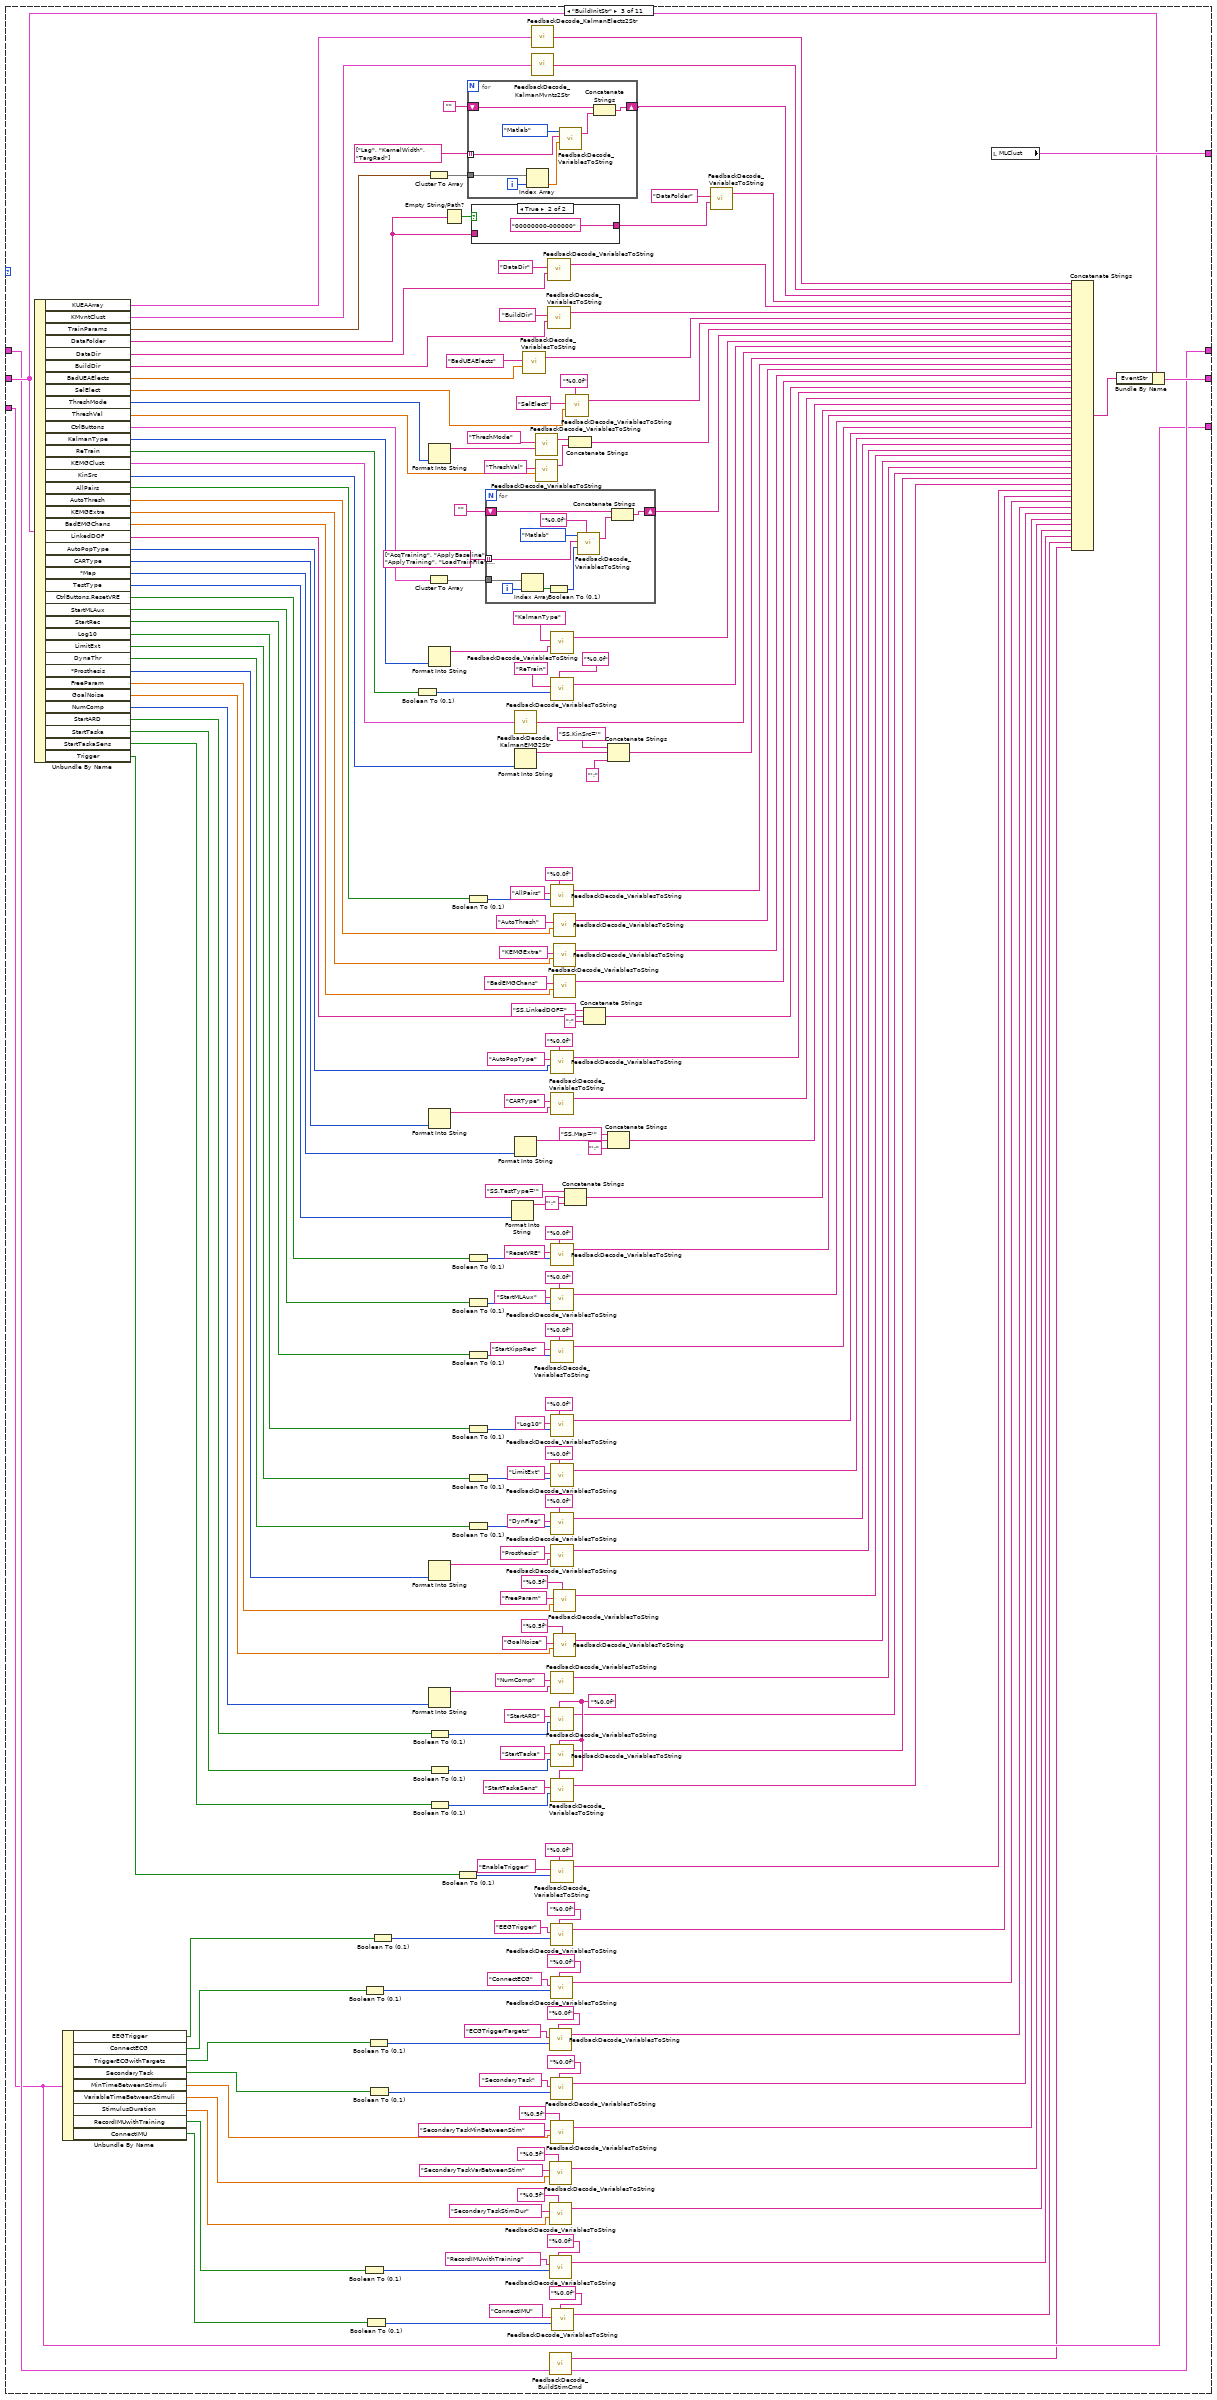
[diagram p5: hidden frame]
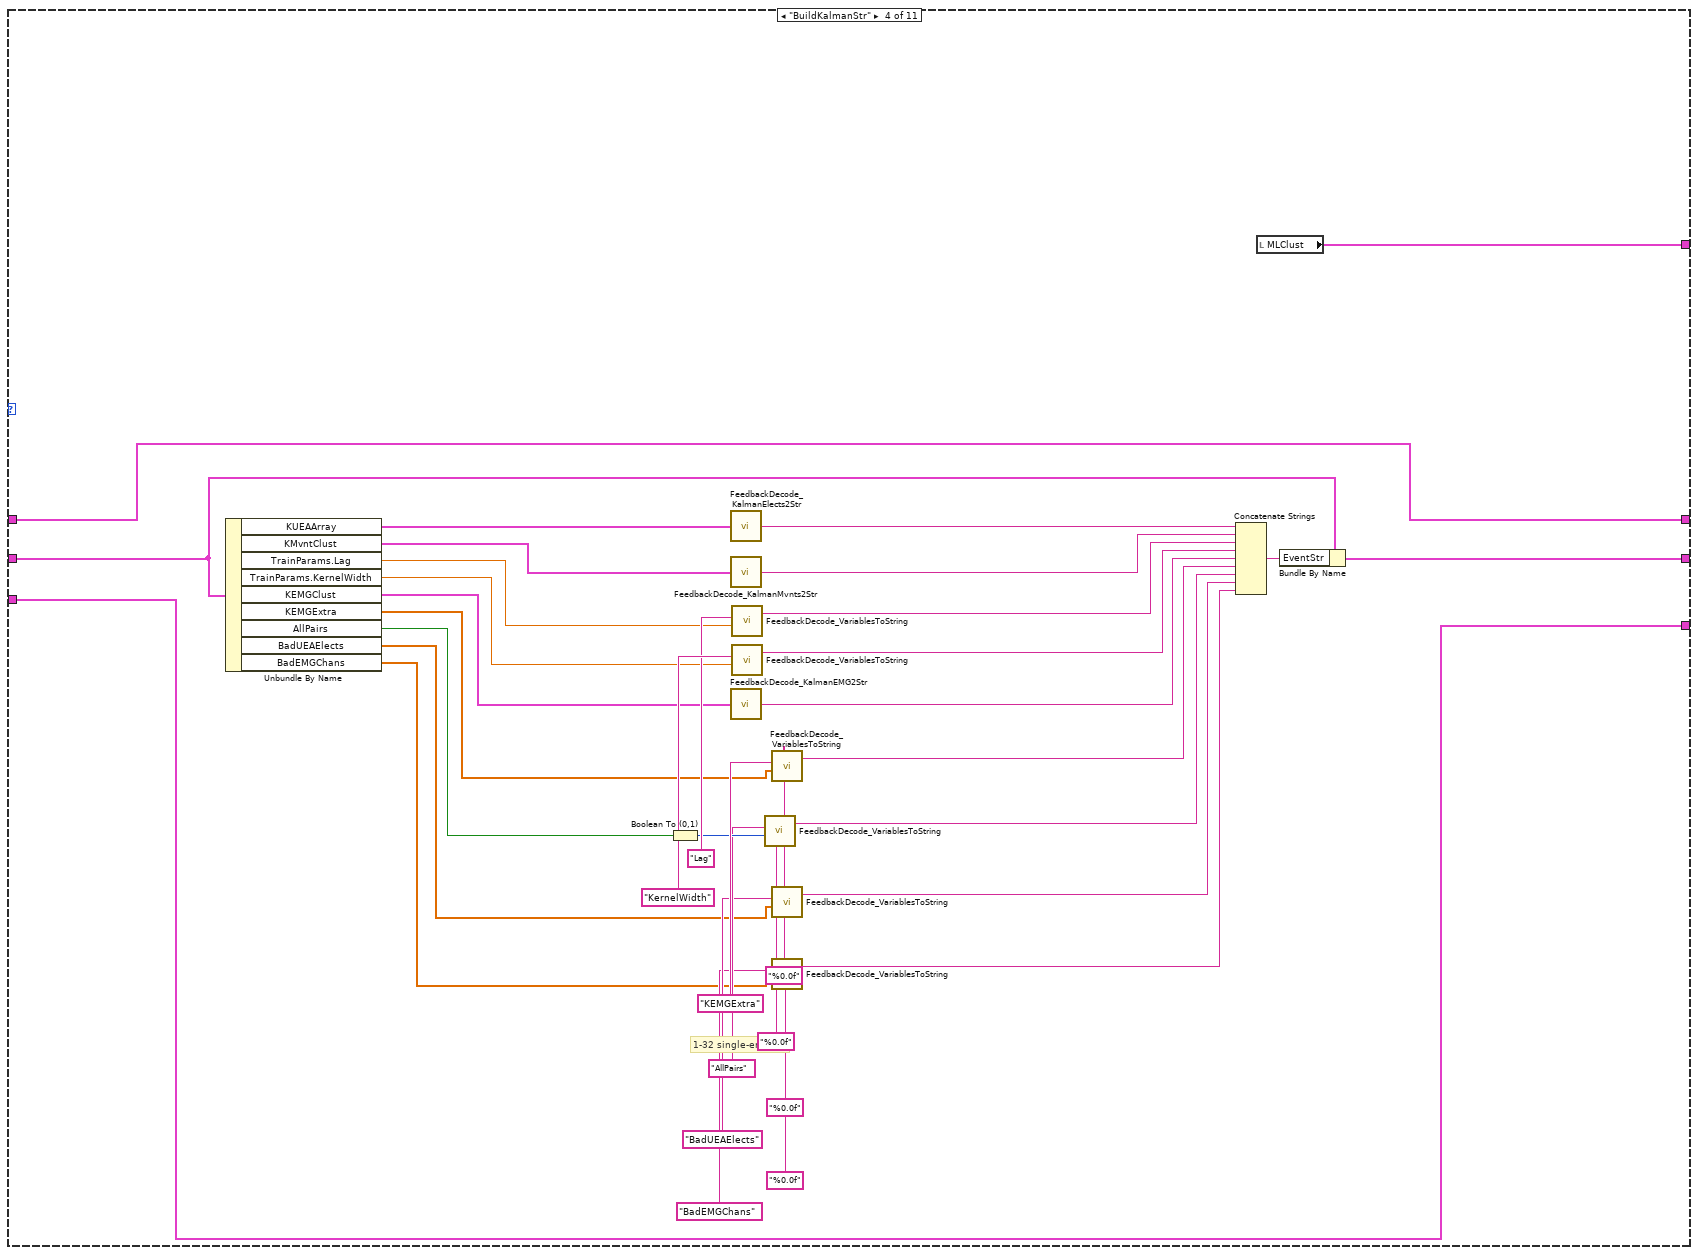
[diagram p7: hidden frame]
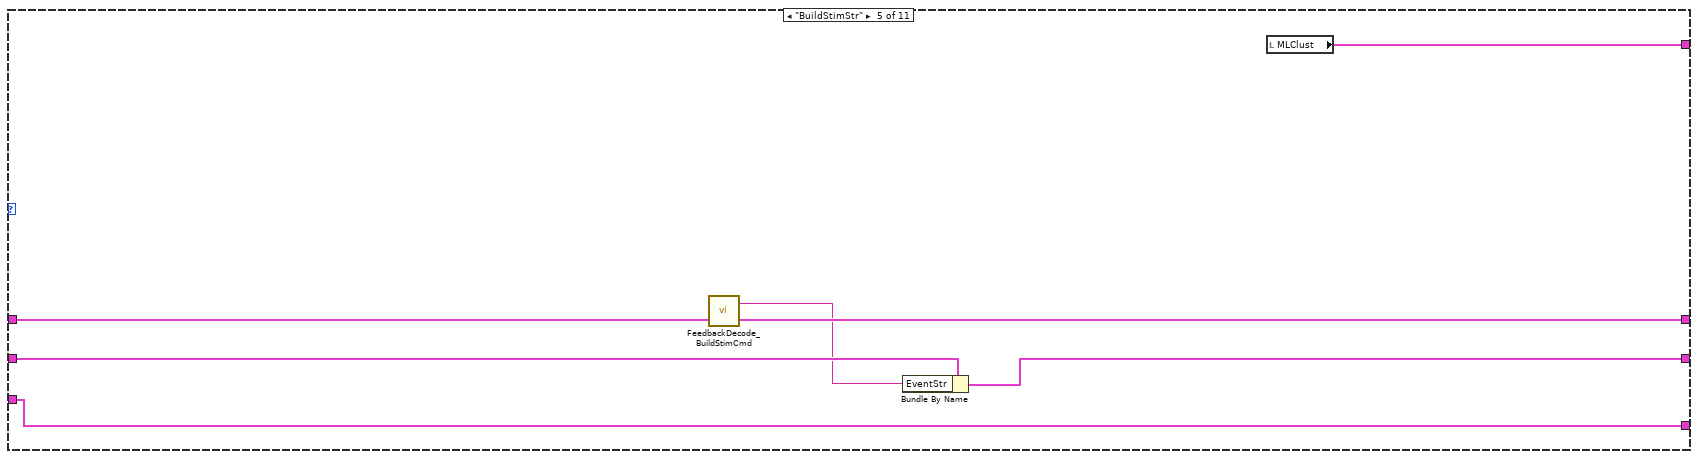
[diagram p8: hidden frame]
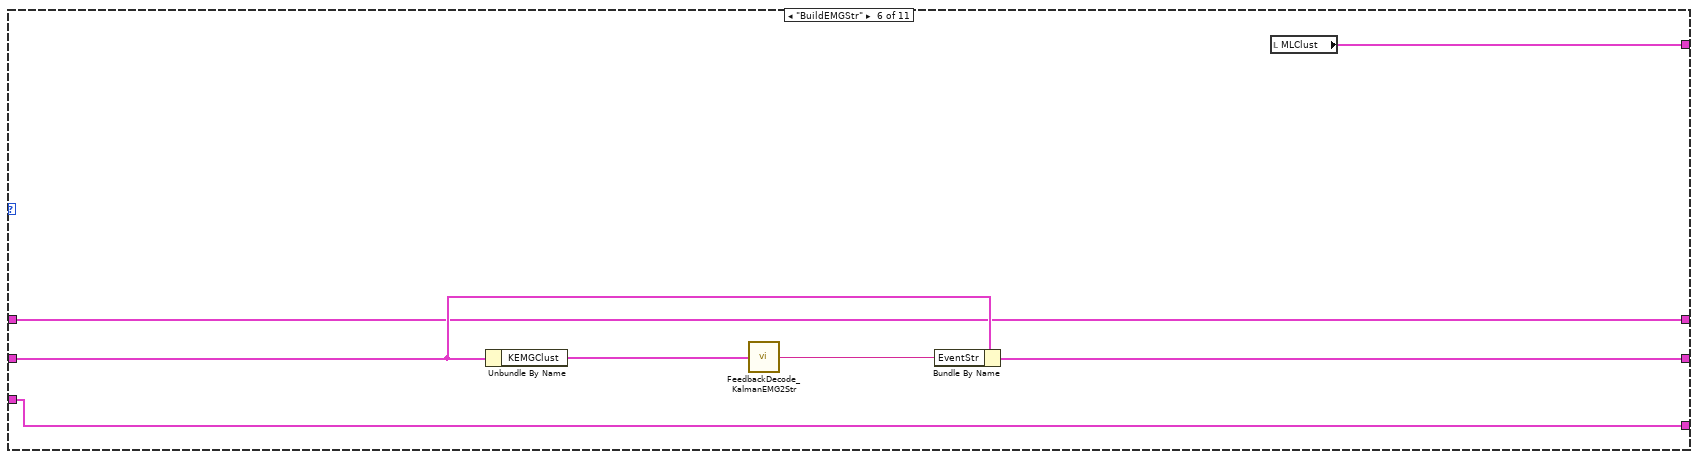
[diagram p9: hidden frame]
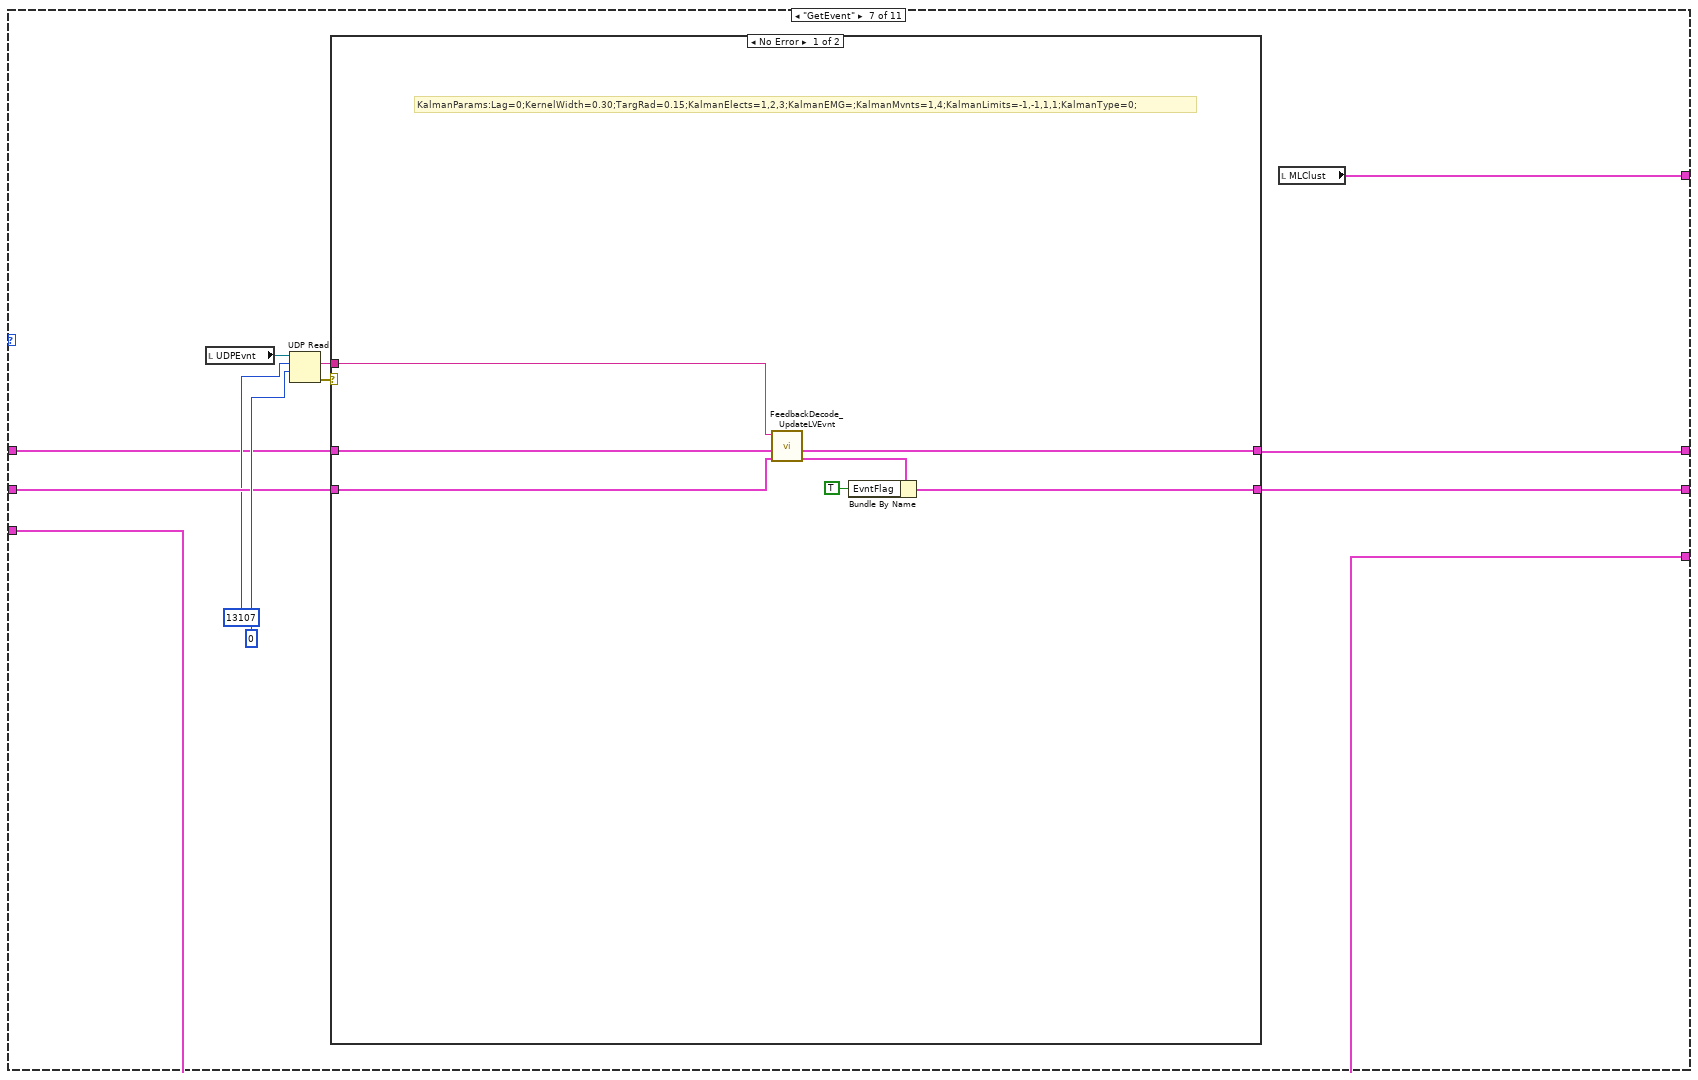
[diagram p10: hidden frame]
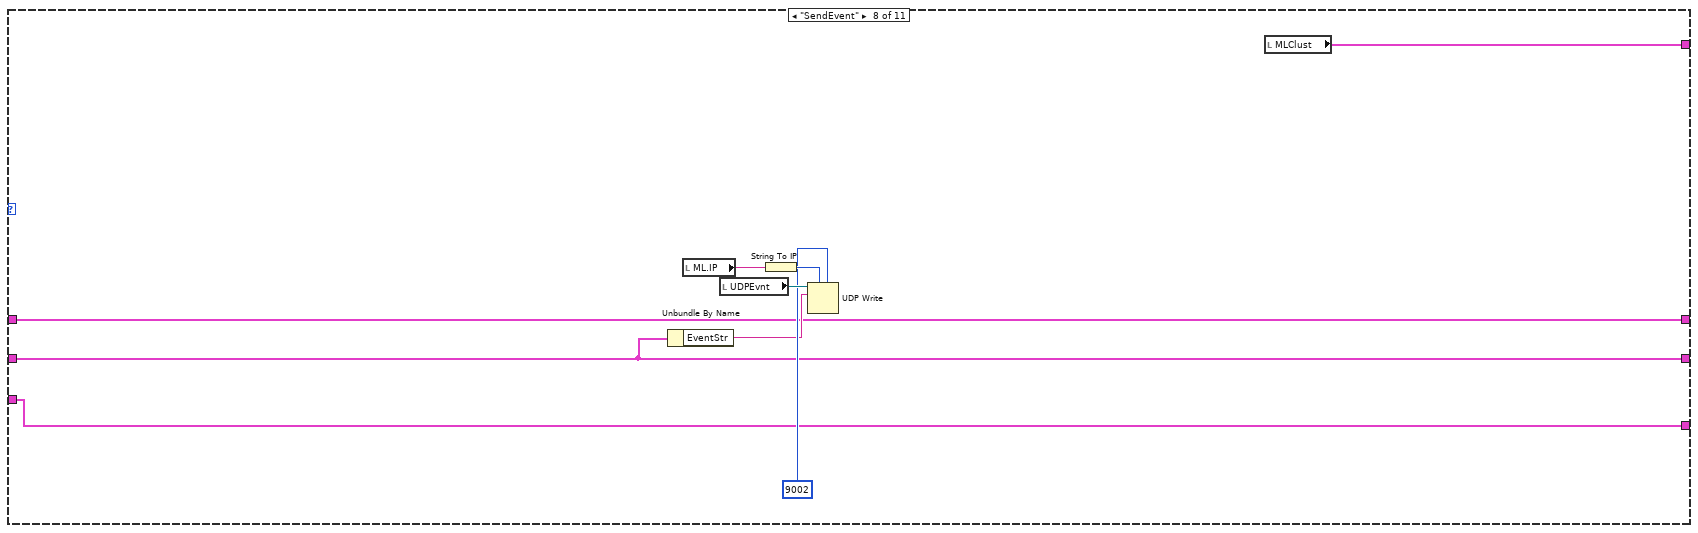
[diagram p12: hidden frame]
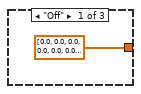
[diagram p13: hidden frame]
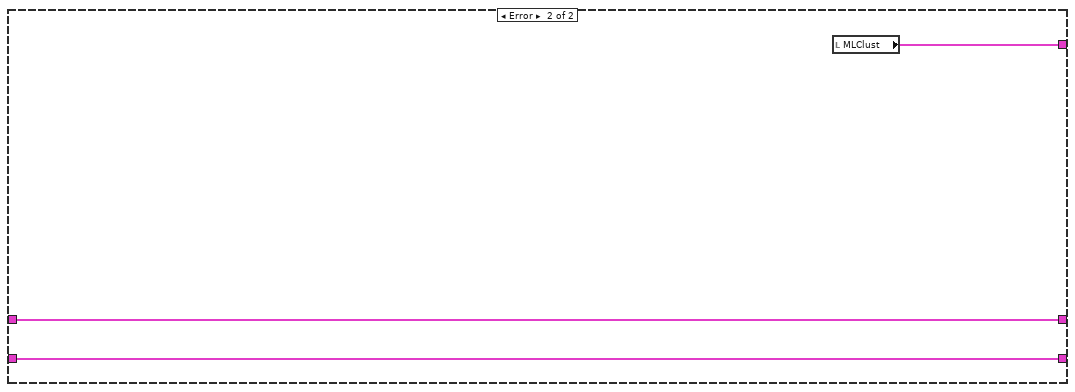
[diagram p15: hidden frame]
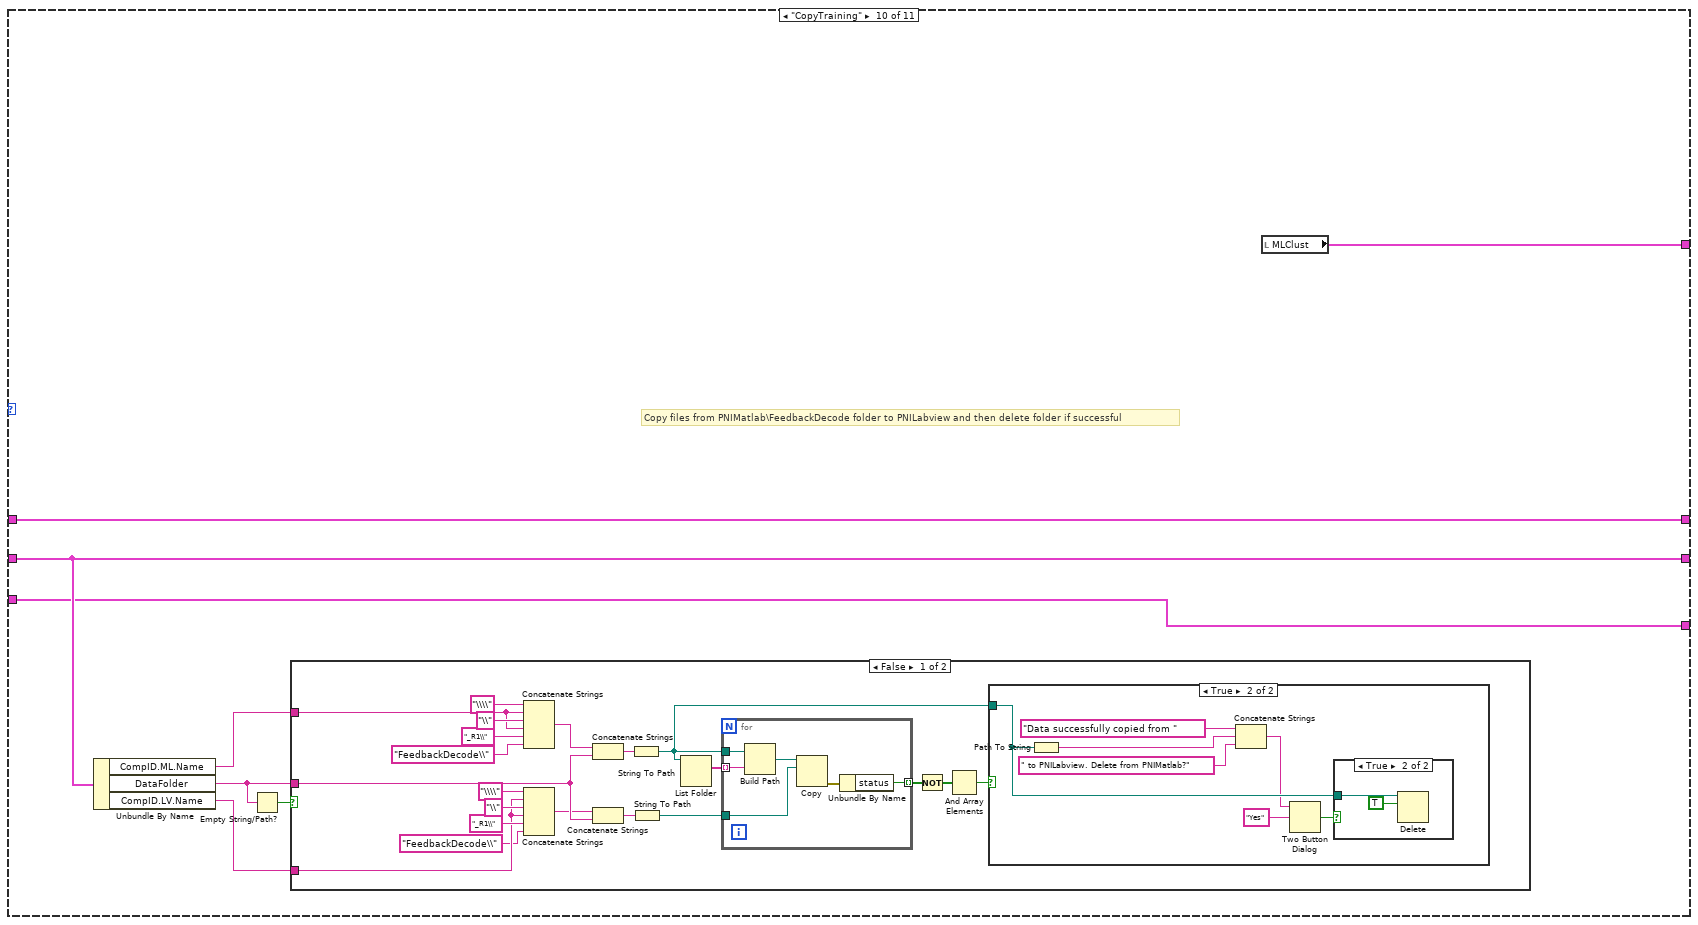
[diagram p16: hidden frame]
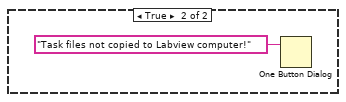
[diagram p19: hidden frame]
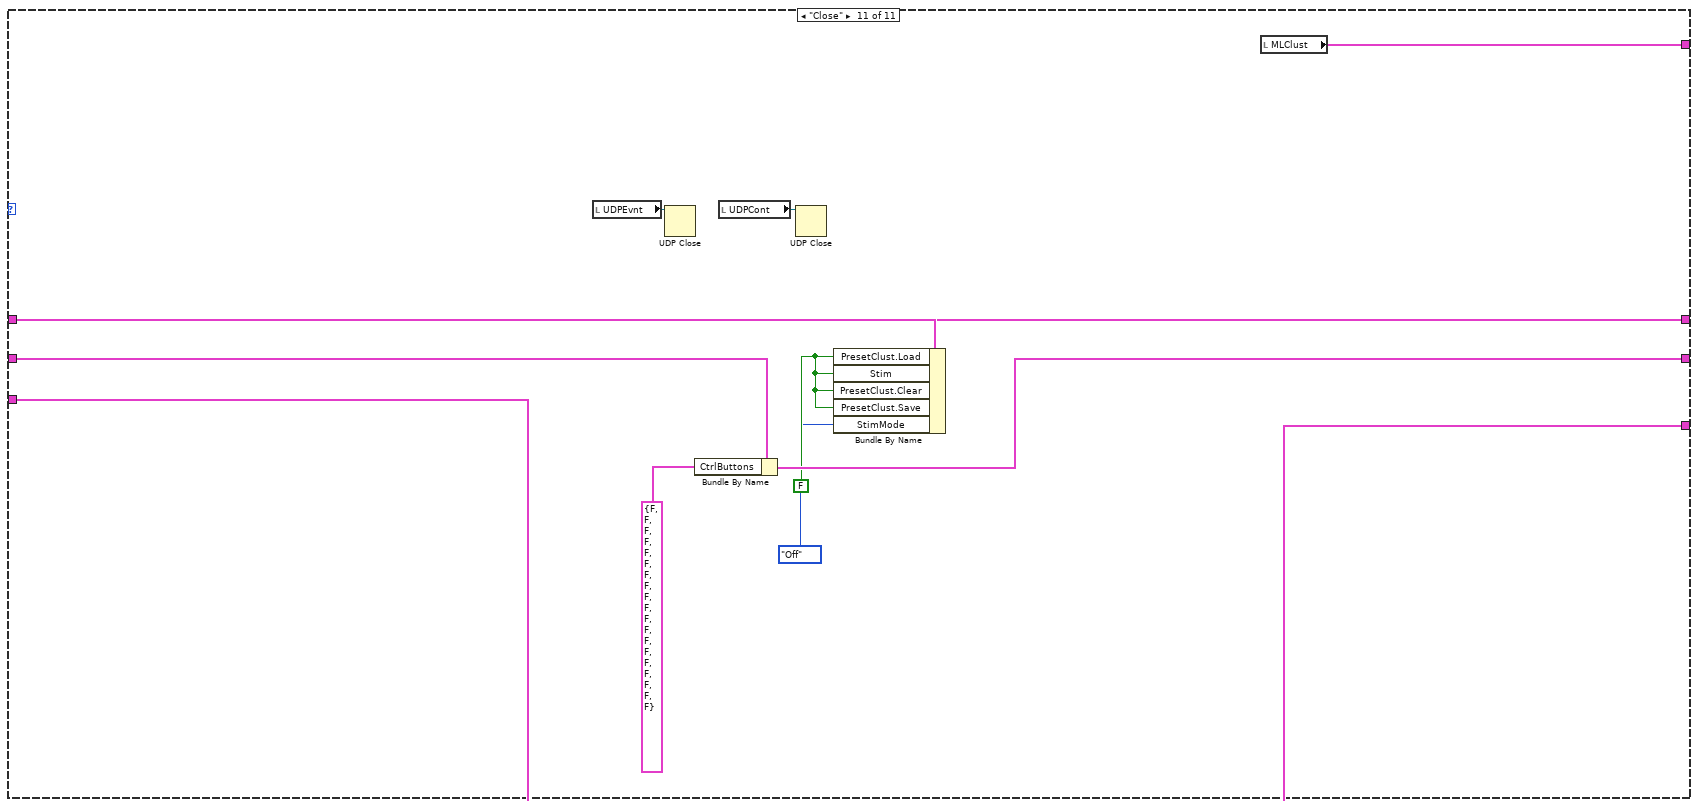
[diagram p20: hidden frame]
diagram:
  n1 = case shown="\"ContIO\"" "Mode" {
    tunnel: "DecodeClustIn" -> [w27 w39 w215 w296 w313 w321 w330 w346 w359 w523 w571]
    tunnel: [w26 w39 w241 w301 w311 w319 w329 w346 w358 w523 w570] -> w5
    tunnel: [w25 w38 w240 w302 w316 w323 w328 w348 w357 w525 w569] -> w7
    tunnel: [w11 w37 w162 w279 w314 w318 w326 w345 w355 w519 w565] -> w3
    tunnel: "EncodeClustIn" -> [w14 w37 w163 w279 w315 w318 w325 w345 w354 w519 w566]
    tunnel: "CognitiveLoadIn" -> [w9 w36 w73 w275 w310 w317 w324 w344 w353 w518 w563]
    tunnel: [w9 w36 w73 w275 w310 w317 w324 w344 w353 w518 w563] -> w1
    frame "Initialize", Default {
      # "Continuous to and from Matlab"
      # "Events to Matlab"
      n2 = Bundle By Name(cluster=w27, "CtrlButtons"=T7 {"AcqTraining"=FALSE, "ApplyBaseline"=FALSE, "ApplyTraining"=FALSE, "LoadTrainFile"=FALSE, "CAR"=FALSE, "NIPSpikes"=FALSE, "AcqBaseline"=FALSE, "Stop"=FALSE, "ResetTrial"=FALSE, "TrialSphrs"=FALSE, "HideSphrs"=FALSE, "StartTrials"=FALSE, "AutoPop"=FALSE, "ResetVRE"=FALSE, "StopVRE"=FALSE, "AcqCAR"=FALSE, "ConARD"=FALSE, "Empty2"=FALSE, "Empty1"=FALSE}) -> (w26:T4)
      n3 = Unbundle By Name(w27) -> ("CompID.ML.IP"=→"ML.IP":string, "CompID.LV.IP"=w28:string)
      "LV.IP" <- w28
      n4 = Unbundle By Name(w14) -> ("SelPreset"=w20:bool[], "Sel"=w17:bool[])
      n5 = Array Size(array=w20) -> (size(s)=w22:i32)
      n6 = Array Size(array=w17) -> (size(s)=w18:i32)
      n7 = Initialize Array(FALSE, w22) -> (w16:bool[])
      n8 = Initialize Array(FALSE, w18) -> (w15:bool[])
      n9 = String To IP(1:w28) -> (0:w35:u32)
      n10 = String To IP(1:w28) -> (0:w30:u32)
      n11 = UDP Open(7:w35, 11:u16 9002 ("port")) -> (port=→"UDPEvnt":refnum<k16>)  [unwired: 3 in, 2 out]
      n12 = UDP Open(7:w30, 11:u16 9005 ("port")) -> (port=→"UDPCont":refnum<k16>)  [unwired: 3 in, 2 out]
      n13 = Bundle By Name(cluster=w14, "SelPreset"=w16, "Sel"=w15, "StimMode"=enum16{"Off", "Manual", "MSMS", "VRE"}."Off", "Stim"=FALSE) -> (w13:T3)
      n14 = call "FeedbackDecode_UpdateParamsTable.vi"("StimClustIn"=w13) -> ("StimClustOut"=w12:T3)  [unwired: 2 in]
      n15 = call "FeedbackDecode_Params2UEA.vi"("StimClustIn"=w12) -> ("StimClustOut"=w11:T3)  [unwired: 2 in]
      n16 = local read "MLClust"() -> (w25:T5)
    }
    frame "Wait" {
      n17 = while {
        stop <- w40 stop-if-true
        n18 = local read "UDPEvnt"() -> (w44:refnum<k16>)
        n19 = UDP Read(connection ID=w44, timeout ms (25000)=1000) -> (data out=w41:string, error out=w42:errorcluster)  [unwired: 2 in, 3 out]
        n20 = case shown="Error" w42 {
          tunnel: w41 -> [w46 _]
          tunnel: [w45 FALSE] -> w40
          frame No Error {
            n21 = Equal?(x=w46, y="MatlabReady") -> (x = y?=w45:bool)
          }
          frame Error {
          }
        }
      }
      n22 = local read "MLClust"() -> (w38:T5)
    }
    frame "BuildInitStr" {
      w52 = "%0.0f" ("Format")
      n23 = Unbundle By Name(w215) -> ("KUEAArray"=w226:T8, "KMvntClust"=w224:T9, "TrainParams"=w254:T10, "DataFolder"=w239:string, "DataDir"=w115:string, "BuildDir"=w112:string, "BadUEAElects"=w191:dbl[], "SelElect"=w245:dbl, "ThreshMode"=w153:T11, "ThreshVal"=w233:dbl, "CtrlButtons"=w228:T12, "KalmanType"=w151:T13, "ReTrain"=w218:bool, "KEMGClust"=w214:T14, "KinSrc"=w212:T15, "AllPairs"=w200:bool, "AutoThresh"=w199:dbl, "KEMGExtra"=w198:dbl[], "BadEMGChans"=w193:dbl[], "LinkedDOF"=w183:string, "AutoPopType"=w187:enum16{"Standard", "Stepwise", "Gram"}, "CARType"=w149:enum16{"Standard", "NN"}, "*Map"=w177:T16, "TestType"=w172:T17, "CtrlButtons.ResetVRE"=w168:bool, "StartMLAux"=w164:bool, "StartRec"=w122:bool, "Log10"=w155:bool, "LimitExt"=w144:bool, "DynaThr"=w135:bool, "*Prosthesis"=w140:enum16{"MaleRight", "MaleLeft"}, "FreeParam"=w132:dbl, "GoalNoise"=w127:dbl, "NumComp"=w118:enum16{"1 Computer", "2 Computers"}, "StartARD"=w55:bool, "StartTaska"=w54:bool, "StartTaskaSens"=w53:bool, "Trigger"=w107:bool)
      n24 = Unbundle By Name(w73) -> ("EEGTrigger"=w105:bool, "ConnectECG"=w104:bool, "TriggerECGwithTargets"=w103:bool, "SecondaryTask"=w102:bool, "MinTimeBetweenStimuli"=w83:dbl, "VariableTimeBetweenStimuli"=w82:dbl, "StimulusDuration"=w81:dbl, "RecordIMUwithTraining"=w66:bool, "ConnectIMU"=w65:bool)
      n25 = Boolean To (0,1)(Boolean=w66) -> (0, 1=w70:i16)
      n26 = Boolean To (0,1)(Boolean=w104) -> (0, 1=w92:i16)
      n27 = Boolean To (0,1)(Boolean=w65) -> (0, 1=w67:i16)
      n28 = Boolean To (0,1)(Boolean=w103) -> (0, 1=w91:i16)
      n29 = Boolean To (0,1)(Boolean=w102) -> (0, 1=w90:i16)
      n30 = Boolean To (0,1)(Boolean=w105) -> (0, 1=w99:i16)
      n31 = Boolean To (0,1)(Boolean=w218) -> (0, 1=w217:i16)
      n32 = Cluster To Array(cluster=w254) -> (array=w250:dbl[])
      n33 = Cluster To Array(cluster=w228) -> (array=w231:bool[])
      n34 = Format Into String(w153) -> (resulting string=w152:string)  [unwired: 3 in, 1 out]
      n35 = Format Into String(w151) -> (resulting string=w150:string)  [unwired: 3 in, 1 out]
      n36 = Format Into String(w149) -> (resulting string=w148:string)  [unwired: 3 in, 1 out]
      n37 = Format Into String(w140) -> (resulting string=w142:string)  [unwired: 3 in, 1 out]
      n38 = Format Into String(w118) -> (resulting string=w119:string)  [unwired: 3 in, 1 out]
      n39 = Boolean To (0,1)(Boolean=w55) -> (0, 1=w61:i16)
      n40 = Boolean To (0,1)(Boolean=w54) -> (0, 1=w58:i16)
      n41 = Boolean To (0,1)(Boolean=w53) -> (0, 1=w57:i16)
      n42 = Empty String/Path?(string/path=w239) -> (empty?=w249:bool)
      n43 = Boolean To (0,1)(Boolean=w107) -> (0, 1=w108:i16)
      n44 = Boolean To (0,1)(Boolean=w200) -> (0, 1=w203:i16)
      n45 = Boolean To (0,1)(Boolean=w168) -> (0, 1=w171:i16)
      n46 = Boolean To (0,1)(Boolean=w164) -> (0, 1=w165:i16)
      n47 = Boolean To (0,1)(Boolean=w122) -> (0, 1=w125:i16)
      n48 = Boolean To (0,1)(Boolean=w155) -> (0, 1=w158:i16)
      n49 = Boolean To (0,1)(Boolean=w144) -> (0, 1=w145:i16)
      n50 = Boolean To (0,1)(Boolean=w135) -> (0, 1=w138:i16)
      n51 = for {
        tunnel: w250 -> [w267]
        tunnel: string[] ["Lag", "KernelWidth", "TargRad"] -> [w269] mode=indexing
        shift-right: [w270] -> w252
        shift-left: "" -> [w271]
        i -> [w273]
        n52 = Index Array(array=w267, index=w273) -> (element=w268:dbl)
        n53 = call-poly "FeedbackDecode_VariablesToString.vi"("ValueIn"=w268, "FieldName"=w269, "Type"=enum16{"Normal", "Matlab"}."Matlab") -> ("StringOut"=w272:string)  [unwired: 4 in]
        n54 = Concatenate Strings(w271, w272) -> (w270:string)
      }
      n55 = case shown="True" w249 {
        tunnel: w239 -> [w265 _]
        tunnel: [w265 "00000000-000000" ("CerebusFolder")] -> w247
        frame False {
        }
        frame True {
        }
      }
      n56 = for {
        tunnel: w231 -> [w258]
        tunnel: string[] ["AcqTraining", "ApplyBaseline", "ApplyTraining", "LoadTrainFile", "CAR", "NIPSpikes", "AcqBaseline", "Stop", "ResetTrial", "CalibrateDEKA", "HideSpheres", "StartTrials", "AutoPop", "ResetVRE", "StopVRE", "AcqCAR", "ConnectARD", "RestartDEKA", "ConnectDEKA"] -> [w259] mode=indexing
        shift-right: [w260] -> w227
        shift-left: "" -> [w261]
        i -> [w263]
        n57 = Index Array(array=w258, index=w263) -> (element=w256:bool)
        n58 = Boolean To (0,1)(Boolean=w256) -> (0, 1=w255:i16)
        n59 = call-poly "FeedbackDecode_VariablesToString.vi"("Format"="%0.0f", "ValueIn"=w255, "FieldName"=w259, "Type"=enum16{"Normal", "Matlab"}."Matlab") -> ("StringOut"=w262:string)  [unwired: 3 in]
        n60 = Concatenate Strings(w261, w262) -> (w260:string)
      }
      n61 = Format Into String(w172) -> (resulting string=w175:string)  [unwired: 3 in, 1 out]
      n62 = call "FeedbackDecode_KalmanEMG2Str.vi"("KalmanEMG"=w214) -> ("KalmanEMGStr"=w213:string)
      n63 = Format Into String(w212) -> (resulting string=w211:string)  [unwired: 3 in, 1 out]
      n64 = Format Into String(w177) -> (resulting string=w178:string)  [unwired: 3 in, 1 out]
      n65 = call-poly "FeedbackDecode_VariablesToString.vi"("ValueIn"=w191, "FieldName"="BadUEAElects") -> ("StringOut"=w206:string)  [unwired: 5 in]
      n66 = call "FeedbackDecode_KalmanElects2Str.vi"("KalmanElects"=w226) -> ("KElectStr"=w225:string)
      n67 = call "FeedbackDecode_KalmanMvnts2Str.vi"("KMvntClust"=w224) -> ("KMvntStr"=w223:string)
      n68 = call-poly "FeedbackDecode_VariablesToString.vi"("ValueIn"=w152, "FieldName"="ThreshMode") -> ("StringOut"=w236:string)  [unwired: 5 in]
      n69 = call-poly "FeedbackDecode_VariablesToString.vi"("ValueIn"=w233, "FieldName"="ThreshVal") -> ("StringOut"=w234:string)  [unwired: 5 in]
      n70 = call-poly "FeedbackDecode_VariablesToString.vi"("ValueIn"=w115, "FieldName"="DataDir") -> ("StringOut"=w114:string)  [unwired: 5 in]
      n71 = call-poly "FeedbackDecode_VariablesToString.vi"("ValueIn"=w112, "FieldName"="BuildDir") -> ("StringOut"=w111:string)  [unwired: 5 in]
      n72 = call-poly "FeedbackDecode_VariablesToString.vi"("Format"="%0.0f", "ValueIn"=w91, "FieldName"="ECGTriggerTargets") -> ("StringOut"=w78:string)  [unwired: 4 in]
      n73 = call-poly "FeedbackDecode_VariablesToString.vi"("Format"="%0.5f", "ValueIn"=w82, "FieldName"="SecondaryTaskVarBetweenStim") -> ("StringOut"=w75:string)  [unwired: 4 in]
      n74 = call-poly "FeedbackDecode_VariablesToString.vi"("Format"="%0.5f", "ValueIn"=w81, "FieldName"="SecondaryTaskStimDur") -> ("StringOut"=w74:string)  [unwired: 4 in]
      n75 = call-poly "FeedbackDecode_VariablesToString.vi"("Format"="%0.0f", "ValueIn"=w70, "FieldName"="RecordIMUwithTraining") -> ("StringOut"=w63:string)  [unwired: 4 in]
      n76 = call "FeedbackDecode_BuildStimCmd.vi"("EncodeClustIn"=w163) -> ("EncodeClustOut"=w162:T3, "StimCmd"=w64:string)  [unwired: 1 in]
      n77 = call-poly "FeedbackDecode_VariablesToString.vi"("Format"="%0.0f", "ValueIn"=w99, "FieldName"="EEGTrigger") -> ("StringOut"=w80:string)  [unwired: 4 in]
      n78 = call-poly "FeedbackDecode_VariablesToString.vi"("Format"="%0.0f", "ValueIn"=w92, "FieldName"="ConnectECG") -> ("StringOut"=w79:string)  [unwired: 4 in]
      n79 = call-poly "FeedbackDecode_VariablesToString.vi"("Format"="%0.0f", "ValueIn"=w90, "FieldName"="SecondaryTask") -> ("StringOut"=w77:string)  [unwired: 4 in]
      n80 = call-poly "FeedbackDecode_VariablesToString.vi"("ValueIn"=w150, "FieldName"="KalmanType") -> ("StringOut"=w221:string)  [unwired: 5 in]
      n81 = call-poly "FeedbackDecode_VariablesToString.vi"("Format"="%0.0f", "ValueIn"=w217, "FieldName"="ReTrain") -> ("StringOut"=w216:string)  [unwired: 4 in]
      n82 = call-poly "FeedbackDecode_VariablesToString.vi"("Format"="%0.0f", "ValueIn"=w203, "FieldName"="AllPairs") -> ("StringOut"=w197:string)  [unwired: 4 in]
      n83 = call-poly "FeedbackDecode_VariablesToString.vi"("Format"="%0.0f", "ValueIn"=w187, "FieldName"="AutoPopType") -> ("StringOut"=w186:string)  [unwired: 4 in]
      n84 = call-poly "FeedbackDecode_VariablesToString.vi"("ValueIn"=w148, "FieldName"="CARType") -> ("StringOut"=w185:string)  [unwired: 5 in]
      n85 = call-poly "FeedbackDecode_VariablesToString.vi"("Format"="%0.0f", "ValueIn"=w171, "FieldName"="ResetVRE") -> ("StringOut"=w160:string)  [unwired: 4 in]
      n86 = call-poly "FeedbackDecode_VariablesToString.vi"("Format"="%0.0f", "ValueIn"=w165, "FieldName"="StartMLAux") -> ("StringOut"=w159:string)  [unwired: 4 in]
      n87 = call-poly "FeedbackDecode_VariablesToString.vi"("Format"="%0.0f", "ValueIn"=w125, "FieldName"="StartXippRec") -> ("StringOut"=w121:string)  [unwired: 4 in]
      n88 = call-poly "FeedbackDecode_VariablesToString.vi"("Format"="%0.0f", "ValueIn"=w158, "FieldName"="Log10") -> ("StringOut"=w154:string)  [unwired: 4 in]
      n89 = call-poly "FeedbackDecode_VariablesToString.vi"("Format"="%0.0f", "ValueIn"=w145, "FieldName"="LimitExt") -> ("StringOut"=w143:string)  [unwired: 4 in]
      n90 = call-poly "FeedbackDecode_VariablesToString.vi"("Format"="%0.0f", "ValueIn"=w138, "FieldName"="DynFlag") -> ("StringOut"=w134:string)  [unwired: 4 in]
      n91 = call-poly "FeedbackDecode_VariablesToString.vi"("ValueIn"=w142, "FieldName"="Prosthesis") -> ("StringOut"=w139:string)  [unwired: 5 in]
      n92 = call-poly "FeedbackDecode_VariablesToString.vi"("ValueIn"=w119, "FieldName"="NumComp") -> ("StringOut"=w117:string)  [unwired: 5 in]
      n93 = call-poly "FeedbackDecode_VariablesToString.vi"("Format"=w52, "ValueIn"=w61, "FieldName"="StartARD") -> ("StringOut"=w51:string)  [unwired: 4 in]
      n94 = call-poly "FeedbackDecode_VariablesToString.vi"("Format"=w52, "ValueIn"=w58, "FieldName"="StartTaska") -> ("StringOut"=w50:string)  [unwired: 4 in]
      n95 = call-poly "FeedbackDecode_VariablesToString.vi"("Format"=w52, "ValueIn"=w57, "FieldName"="StartTaskaSens") -> ("StringOut"=w49:string)  [unwired: 4 in]
      n96 = call-poly "FeedbackDecode_VariablesToString.vi"("Format"="%0.0f", "ValueIn"=w108, "FieldName"="EnableTrigger") -> ("StringOut"=w106:string)  [unwired: 4 in]
      n97 = call-poly "FeedbackDecode_VariablesToString.vi"("Format"="%0.5f", "ValueIn"=w83, "FieldName"="SecondaryTaskMinBetweenStim") -> ("StringOut"=w76:string)  [unwired: 4 in]
      n98 = call-poly "FeedbackDecode_VariablesToString.vi"("Format"="%0.0f", "ValueIn"=w67, "FieldName"="ConnectIMU") -> ("StringOut"=w62:string)  [unwired: 4 in]
      n99 = call-poly "FeedbackDecode_VariablesToString.vi"("ValueIn"=w199, "FieldName"="AutoThresh") -> ("StringOut"=w196:string)  [unwired: 5 in]
      n100 = call-poly "FeedbackDecode_VariablesToString.vi"("ValueIn"=w198, "FieldName"="KEMGExtra") -> ("StringOut"=w195:string)  [unwired: 5 in]
      n101 = call-poly "FeedbackDecode_VariablesToString.vi"("ValueIn"=w193, "FieldName"="BadEMGChans") -> ("StringOut"=w192:string)  [unwired: 5 in]
      n102 = call-poly "FeedbackDecode_VariablesToString.vi"("Format"="%0.5f", "ValueIn"=w132, "FieldName"="FreeParam") -> ("StringOut"=w130:string)  [unwired: 4 in]
      n103 = call-poly "FeedbackDecode_VariablesToString.vi"("Format"="%0.5f", "ValueIn"=w127, "FieldName"="GoalNoise") -> ("StringOut"=w126:string)  [unwired: 4 in]
      n104 = Concatenate Strings("SS.TestType='" ("string"), w175, "';" ("string")) -> (w161:string)
      n105 = call-poly "FeedbackDecode_VariablesToString.vi"("Format"="%0.0f", "ValueIn"=w245, "FieldName"="SelElect") -> ("StringOut"=w244:string)  [unwired: 4 in]
      n106 = Concatenate Strings(w236, w234) -> (w232:string)
      n107 = Concatenate Strings("SS.LinkedDOF=" ("FieldName"), w183, ";" ("string")) -> (w182:string)
      n108 = Concatenate Strings("SS.KinSrc='" ("string"), w211, "';" ("string")) -> (w208:string)
      n109 = Concatenate Strings("SS.Map='" ("string"), w178, "';" ("string")) -> (w176:string)
      n110 = call-poly "FeedbackDecode_VariablesToString.vi"("ValueIn"=w247, "FieldName"="DataFolder") -> ("StringOut"=w238:string)  [unwired: 5 in]
      n111 = local read "MLClust"() -> (w240:T5)
      n112 = Concatenate Strings(w225, w223, w252, w238, w114, w111, w206, w244, w232, w227, w221, w216, w213, w208, w197, w196, w195, w192, w182, w186, w185, w176, w161, w160, w159, w121, w154, w143, w134, w139, w130, w126, w117, w51, w50, w49, w106, w80, w79, w78, w77, w76, w75, w74, w63, w62, w64) -> (w242:string)
      n113 = Bundle By Name(cluster=w215, "EventStr"=w242) -> (w241:T4)
    }
    frame "BuildKalmanStr" {
      # "1-32 single-ended"
      n114 = Unbundle By Name(w296) -> ("KUEAArray"=w300:T8, "KMvntClust"=w298:T9, "TrainParams.Lag"=w305:dbl, "TrainParams.KernelWidth"=w304:dbl, "KEMGClust"=w294:T14, "KEMGExtra"=w292:dbl[], "AllPairs"=w287:bool, "BadUEAElects"=w280:dbl[], "BadEMGChans"=w283:dbl[])
      n115 = Boolean To (0,1)(Boolean=w287) -> (0, 1=w290:i16)
      n116 = call "FeedbackDecode_KalmanElects2Str.vi"("KalmanElects"=w300) -> ("KElectStr"=w299:string)
      n117 = call "FeedbackDecode_KalmanMvnts2Str.vi"("KMvntClust"=w298) -> ("KMvntStr"=w297:string)
      n118 = call "FeedbackDecode_KalmanEMG2Str.vi"("KalmanEMG"=w294) -> ("KalmanEMGStr"=w295:string)
      n119 = call-poly "FeedbackDecode_VariablesToString.vi"("ValueIn"=w305, "FieldName"="Lag" ("Key Word")) -> ("StringOut"=w307:string)  [unwired: 5 in]
      n120 = call-poly "FeedbackDecode_VariablesToString.vi"("ValueIn"=w304, "FieldName"="KernelWidth" ("Key Word")) -> ("StringOut"=w306:string)  [unwired: 5 in]
      n121 = call-poly "FeedbackDecode_VariablesToString.vi"("Format"="%0.0f", "ValueIn"=w290, "FieldName"="AllPairs") -> ("StringOut"=w286:string)  [unwired: 4 in]
      n122 = call-poly "FeedbackDecode_VariablesToString.vi"("Format"="%0.0f", "ValueIn"=w292, "FieldName"="KEMGExtra") -> ("StringOut"=w291:string)  [unwired: 4 in]
      n123 = call-poly "FeedbackDecode_VariablesToString.vi"("Format"="%0.0f", "ValueIn"=w280, "FieldName"="BadUEAElects") -> ("StringOut"=w282:string)  [unwired: 4 in]
      n124 = call-poly "FeedbackDecode_VariablesToString.vi"("Format"="%0.0f", "ValueIn"=w283, "FieldName"="BadEMGChans") -> ("StringOut"=w281:string)  [unwired: 4 in]
      n125 = Concatenate Strings(w299, w297, w307, w306, w295, w291, w286, w282, w281) -> (w303:string)
      n126 = local read "MLClust"() -> (w302:T5)
      n127 = Bundle By Name(cluster=w296, "EventStr"=w303) -> (w301:T4)
    }
    frame "BuildStimStr" {
      n128 = call "FeedbackDecode_BuildStimCmd.vi"("EncodeClustIn"=w315) -> ("EncodeClustOut"=w314:T3, "StimCmd"=w312:string)  [unwired: 1 in]
      n129 = Bundle By Name(cluster=w313, "EventStr"=w312) -> (w311:T4)
      n130 = local read "MLClust"() -> (w316:T5)
    }
    frame "BuildEMGStr" {
      n131 = Unbundle By Name(w321) -> ("KEMGClust"=w322:T14)
      n132 = call "FeedbackDecode_KalmanEMG2Str.vi"("KalmanEMG"=w322) -> ("KalmanEMGStr"=w320:string)
      n133 = Bundle By Name(cluster=w321, "EventStr"=w320) -> (w319:T4)
      n134 = local read "MLClust"() -> (w323:T5)
    }
    frame "GetEvent" {
      n135 = local read "UDPEvnt"() -> (w334:refnum<k16>)
      n136 = UDP Read(connection ID=w334, max size (548)=13107 ("timeout ms (25000)"), timeout ms (25000)=0) -> (data out=w331:string, error out=w332:errorcluster)  [unwired: 1 in, 3 out]
      n137 = case shown="No Error" w332 {
        tunnel: w331 -> [w339 _]
        tunnel: w330 -> [w338 w343]
        tunnel: [w340 w343] -> w329
        tunnel: [w335 w342] -> w326
        tunnel: w325 -> [w337 w342]
        frame No Error {
          # "KalmanParams:Lag=0;KernelWidth=0.30;TargRad=0.15;KalmanElects=1,2,3;KalmanEMG=;KalmanMvnts=1,4;KalmanLimits=-1,-1,1,1;KalmanType=0;"
          n138 = call "FeedbackDecode_UpdateLVEvnt.vi"("DecodeClustIn"=w338, "EncodeClustIn"=w337, "EvntStrIn"=w339) -> ("DecodeClustOut"=w336:T4, "EncodeClustOut"=w335:T3)  [unwired: 3 in]
          n139 = Bundle By Name(cluster=w336, "EvntFlag"=TRUE) -> (w340:T4)
        }
        frame Error {
        }
      }
      n140 = local read "MLClust"() -> (w328:T5)
    }
    frame "SendEvent" {
      n141 = Unbundle By Name(w346) -> ("EventStr"=w347:string)
      n142 = local read "ML.IP"() -> (w349:string)
      n143 = local read "UDPEvnt"() -> (w352:refnum<k16>)
      n144 = String To IP(1:w349) -> (0:w351:u32)
      n145 = UDP Write(address=w351, port or service name=u16 9002 ("port"), connection ID=w352, data in=w347) -> ()  [unwired: 2 in, 2 out]
      n146 = local read "MLClust"() -> (w348:T5)
    }
    frame "ContIO" {
      n147 = local read "UDPCont"() -> (w364:refnum<k16>)
      n148 = UDP Read(connection ID=w364, max size (548)=13107 ("timeout ms (25000)"), timeout ms (25000)=0) -> (data out=w362:string, error out=w360:errorcluster, 3:w356:refnum<k16>)  [unwired: 1 in, 2 out]
      n149 = case shown="No Error" w360 {
        selector: w360 -> [w462 _]
        tunnel: w362 -> [w505 _]
        tunnel: w359 -> [w452 w516]
        tunnel: [w452 w516] -> w358
        tunnel: [w489 w517] -> w357
        tunnel: w356 -> [w463 _]
        tunnel: [w400 w515] -> w355
        tunnel: w354 -> [w400 w515]
        frame No Error {
          w365 = 4 ("length")
          w367 = 12 ("length")
          w376 = 13 ("length")
          w379 = 52 ("length")
          w382 = 1 ("length")
          w392 = 1 ("length")
          w456 = 80 ("length")
          w397 = 48 ("length")
          w480 = 1 ("length")
          w482 = 1 ("length")
          w483 = 28 ("index")
          # "TASKA Baro"
          # "TASKA IR"
          # "raw decode\noutput"
          # "stim wf"
          # "deka sensors"
          # "TrainCount\nMLCalcTime\nMLTotalTime\nKalman (xhat, 12)\nKinematics (x, 12)\nElectRate (length, 1)\nElectRates (above length)\nSelThresh (scalar)\nSelData (length, 1)\nSelData (above length)\nSelWf (48)\nNIPTime(1)\nVREID(1)\nStimWF(52)\nDEKAsensors(13) - global\nrawDecodeOutput(12) - global\ntaska IR sensors (3)\ntaska baro sensors (3)"
          # "EMGPwr"
          # "SelWf"
          # "Length ElectRates"
          # "Only taking first wf from selected electrode each loop iteration to reduce matlab calc time"
          # "SelData"
          # "Length SelData"
          # "SelThresh"
          # "ElectRates"
          # "Kinematics"
          # "Kalman"
          # "Loop times"
          n150 = Unbundle By Name(w452) -> ("RasterWin"=w431:dbl, "SelElect"=w433:dbl, "Kinematics"=w421:T18, "KinSrc"=w418:T15)
          n151 = call "FeedbackDecode_UDPStr2Single.vi"("UDPStr"=w505) -> ("UDPSingle"=w371:sgl[])
          n152 = Cluster To Array(cluster=w421) -> (array=w420:dbl[])
          n153 = Array Subset(array=w371, index=0, length=1) -> (w476:sgl[])
          n154 = Array Subset(array=w371, index=1, length=2) -> (w495:sgl[])
          n155 = Array Subset(array=w371, index=3, length=12) -> (w416:sgl[])
          n156 = Array Subset(array=w371, index=15, length=12) -> (w419:sgl[])
          n157 = Array Subset(array=w371, index=27, length=1) -> (w487:sgl[])
          n158 = Array To Cluster(array=w495) -> (cluster=w494:cluster{"[0]":sgl, "[1]":sgl})
          n159 = Index Array(array=w476) -> (element=w458:sgl)  [unwired: 1 in]
          n160 = Array To Cluster(array=w419) -> (cluster=w492:T19)
          n161 = Array To Cluster(array=w416) -> (cluster=w493:T19)
          n162 = Index Array(array=w487) -> (element=w484:sgl)  [unwired: 1 in]
          n163 = Add(x=w484, y=w483) -> (x+y=w457:sgl)
          n164 = Add(x=w457, y=w456) -> (x+y=w455:sgl)
          n165 = Add(x=w455, y=w482) -> (x+y=w481:sgl)
          n166 = Add(x=w481, y=w480) -> (x+y=w479:sgl)
          n167 = Array Subset(array=w371, index=w483, length=w484) -> (w435:sgl[])
          n168 = Array Subset(array=w371, index=w457, length=w456) -> (w436:sgl[])
          n169 = Array Subset(array=w371, index=w455, length=w482) -> (w444:sgl[])
          n170 = Array Subset(array=w371, index=w481, length=w480) -> (w491:sgl[])
          n171 = Index Array(array=w491) -> (element=w490:sgl)  [unwired: 1 in]
          n172 = Build Array (concatenate)(w420, w419) -> (w417:dbl[])
          n173 = case shown="\"Decode\", Default" w418 {
            tunnel: w417 -> [_ w511 _]
            tunnel: w416 -> [_ _ w514]
            tunnel: [dbl[] [0.0, 0.0, 0.0, 0.0, 0.0, 0.0, 0.0, 0.0, 0.0, 0.0, 0.0, 0.0, 0.0, 0.0, 0.0, 0.0, 0.0, 0.0, 0.0, 0.0, 0.0, 0.0, 0.0, 0.0] w511 w512] -> w415
            frame "Off" {
            }
            frame "Training" {
            }
            frame "Decode", Default {
              n174 = Build Array (concatenate)(w514, dbl[] [0.0, 0.0, 0.0, 0.0, 0.0, 0.0, 0.0, 0.0, 0.0, 0.0, 0.0, 0.0]) -> (w512:dbl[])
            }
          }
          n175 = Decrement(x=w433) -> (x-1=w432:dbl)
          n176 = expression code="floor(x/0.033)*2"(w431) -> (w441:dbl)
          n177 = global read "FeedbackDecode_Globals.vi" "FD_Sensors"() -> (w390:T20)
          n178 = expression code="floor(x/0.033)"(w431) -> (w411:dbl)
          n179 = Build Array (concatenate)(w435, w436) -> (w434:sgl[])
          n180 = Add(x=w479, y=w490) -> (x+y=w398:sgl)
          n181 = Add(x=w398, y=w397) -> (x+y=w393:sgl)
          n182 = Add(x=w393, y=w392) -> (x+y=w383:sgl)
          n183 = Add(x=w383, y=w382) -> (x+y=w378:sgl)
          n184 = Add(x=w378, y=w379) -> (x+y=w375:sgl)
          n185 = Add(x=w375, y=w376) -> (x+y=w368:sgl)
          n186 = Add(x=w368, y=w367) -> (x+y=w366:sgl)
          n187 = Add(x=w366, y=w365) -> (x+y=w373:sgl)
          n188 = Array Subset(array=w371, index=w398, length=w397) -> (w399:sgl[])
          n189 = Array Subset(array=w371, index=w393, length=w392) -> (w396:sgl[])
          n190 = Array Subset(array=w371, index=w383, length=w382) -> (w394:sgl[])
          n191 = Array Subset(array=w371, index=w378, length=w379) -> (w381:sgl[])
          n192 = Array Subset(array=w371, index=w375, length=w376) -> (w377:sgl[])
          n193 = Array Subset(array=w371, index=w368, length=w367) -> (w374:sgl[])
          n194 = Array Subset(array=w371, index=w366, length=w365) -> (w370:sgl[])
          n195 = Array Subset(array=w371, index=w373, length=4) -> (w369:sgl[])
          n196 = Index Array(array=w396) -> (element=w395:sgl)  [unwired: 1 in]
          n197 = Index Array(array=w394) -> (element=w391:sgl)  [unwired: 1 in]
          n198 = global write "FeedbackDecode_Globals.vi" "FD_DEKAsensors"(w377) -> ()
          n199 = Array Subset(array=w371, index=w479, length=w490) -> (w453:sgl[])
          n200 = Build Array (concatenate)(w444, w444) -> (w443:sgl[])
          n201 = Index Array(array=w434, index=w432) -> (element=w424:sgl)
          n202 = Unbundle By Name(w452) -> ("Kinematics"=w465:T18, "Targets"=w464:T18, "State"=w461:T21, "TargDist"=w460:dbl[])
          n203 = Build Array(w453) -> (w454:sgl[][])
          n204 = Unbundle By Name(w390) -> ("Force"=w388:T22, "Position"=w387:T23)
          n205 = Build Array(w424) -> (w423:sgl[])
          n206 = call "FeedbackDecode_CustomRaster.vi"("StitchArray"=w454, "RBuffSize"=w441) -> ("CurIdx"=w439:i32, "RasterOut"=w445:dbl[][])  [unwired: 5 in]
          n207 = Build Array(w423) -> (w422:sgl[][])
          n208 = Build Array(w415) -> (w414:dbl[][])
          n209 = global read "FeedbackDecode_Globals.vi" "FD_Force"() -> (w380:dbl[])
          n210 = Index Array(array=w445) -> (element=w451:dbl[])  [unwired: 2 in]
          n211 = Cluster To Array(cluster=w388) -> (array=w389:dbl[])
          n212 = Cluster To Array(cluster=w387) -> (array=w386:dbl[])
          n213 = call "FeedbackDecode_GenContStimFreq.vi"("EncodeClust"=w400, "TargDist"=w460, "State"=w461) -> ("ContStimFreq"=w459:dbl[])  [unwired: 2 in]
          n214 = Cluster To Array(cluster=w465) -> (array=w468:dbl[])
          n215 = Cluster To Array(cluster=w464) -> (array=w467:dbl[])
          n216 = Cluster To Array(cluster="ManualDOF") -> (array=w384:enum8{"False", "True", "Mixed"}[])
          n217 = Transpose 2D Array(2D array=w414) -> (transposed array=w413:dbl[][])
          n218 = call "FeedbackDecode_CustomRaster.vi"("StitchArray"=w422, "RBuffSize"=w411) -> ("CurIdx"=w409:i32, "RasterOut"=w430:dbl[][])  [unwired: 5 in]
          n219 = Bundle("CurIdx"=w439, 0.0, dbl[] [-250.0, 250.0]) -> (w437:cluster{"CurIdx":i32, dbl, dbl[]})  [unwired: 1 in]
          n220 = call "FeedbackDecode_CustomRaster.vi"("StitchArray"=w413, "RBuffSize"=w411) -> ("CurIdx"=w404:i32, "RasterOut"=w412:dbl[][])  [unwired: 5 in]
          n221 = Index Array(array=w430) -> (element=w427:dbl[])  [unwired: 2 in]
          n222 = Build Array (concatenate)(w468, w467, w459, w389, w386, w384, w380) -> (w466:dbl[])
          n223 = Unbundle By Name(w452) -> ("WfCnt"=w478:dbl, "ClearWfs"=w477:bool)
          n224 = for {
            tunnel: [w507] -> w402 mode=indexing
            tunnel: w412 -> [w506] mode=indexing
            n225 = Bundle(0.0, 1.0, "RasterOut"=w506) -> (w507:cluster{dbl, dbl, "RasterOut":dbl[]})  [unwired: 1 in]
          }
          n226 = To Single Precision Float(number=w466) -> (single precision float=w469:sgl[])
          n227 = Bundle(0.0, 1.0, "RasterOut"=w451) -> (w449:cluster{dbl, dbl, "RasterOut":dbl[]})  [unwired: 1 in]
          n228 = local read "ML.IP"() -> (w472:string)
          n229 = Bundle(0.0, 1.0, "RasterOut"=w427) -> (w426:cluster{dbl, dbl, "RasterOut":dbl[]})  [unwired: 1 in]
          n230 = Type Cast(type=u8[] [], x=w469) -> (*(type *) &x=w474:u8[])
          n231 = Bundle("CurIdx"=w404, 0.0, dbl[] [-1.0, 1.0]) -> (w401:cluster{"CurIdx":i32, dbl, dbl[]})  [unwired: 1 in]
          n232 = Bundle(0.0, "RasterWin"=w441, w443) -> (w450:cluster{dbl, "RasterWin":dbl, sgl[]})  [unwired: 1 in]
          n233 = Bundle("CurIdx"=w409, 0.0, dbl[] [0.0, 120.0]) -> (w405:cluster{"CurIdx":i32, dbl, dbl[]})  [unwired: 1 in]
          n234 = Byte Array To String(unsigned byte array=w474) -> (string=w473:string)
          n235 = call "FeedbackDecode_GenWfBuff.vi"("ClearWfs"=w477, "WfCnt"=w478, "Wf"=w399) -> ("WfBuff"=w488:dbl[][])
          n236 = String To IP(1:w472) -> (0:w470:u32)
          n237 = UDP Write(address=w470, port or service name=u16 9005 ("port"), connection ID=w463, data in=w473, 8:w462) -> ()  [unwired: 1 in, 2 out]
          n238 = Build Array(w437, w450, w449) -> (w442:T24)
          n239 = Build Array(w405, w426) -> (w425:cluster{"CurIdx":dbl, dbl, "RasterOut":dbl[]}[])
          n240 = Build Array (concatenate)(w402, w401) -> (w403:cluster{"CurIdx":dbl, dbl, "RasterOut":dbl[]}[])
          n241 = local read "MLClust"() -> (w496:T5)
          n242 = Bundle By Name(cluster=w496, "TrainCnt"=w458, "LoopTimings"=w494, "Kalman"=w493, "Kinematics"=w492, "ElectRates"=w435, "EMGPwr"=w436, "SelWfs"=w488, "SelData"=w442, "SelRate"=w425, "SelKin"=w403, "NIPTime"=w395, "VREID"=w391, "StimWf"=w381, "RawDecodeOutput"=w374, "TASKA IR sensors"=w370, "TASKA baro sensors"=w369) -> (w489:T5)
        }
        frame Error {
          n243 = local read "MLClust"() -> (w517:T5)
        }
      }
    }
    frame "CopyTraining" {
      # "Copy files from PNIMatlab\\FeedbackDecode folder to PNILabview and then delete folder if successful"
      n244 = Unbundle By Name(w523) -> ("CompID.ML.Name"=w522:string, "DataFolder"=w520:string, "CompID.LV.Name"=w521:string)
      n245 = Empty String/Path?(string/path=w520) -> (empty?=w524:bool)
      n246 = case shown="False" w524 {
        tunnel: w520 -> [w542 _]
        tunnel: w522 -> [w532 _]
        tunnel: w521 -> [w531 _]
        frame False {
          n247 = Concatenate Strings("\\\\" ("string"), w532, "\\" ("string"), w532, "_R1\\" ("string"), "FeedbackDecode\\" ("string")) -> (w533:string)
          n248 = Concatenate Strings("\\\\" ("string"), w531, "\\" ("string"), w531, "_R1\\" ("string"), "FeedbackDecode\\" ("string")) -> (w535:string)
          n249 = Concatenate Strings(w533, w542) -> (w546:string)
          n250 = Concatenate Strings(w535, w542) -> (w545:string)
          n251 = String To Path(string=w546) -> (path=w528:path)
          n252 = String To Path(string=w545) -> (path=w544:path)
          n253 = List Folder(path=w528) -> (filenames=w543:string[])  [unwired: 3 in, 3 out]
          n254 = for {
            tunnel: w544 -> [w561]
            tunnel: w528 -> [w560]
            tunnel: w543 -> [w559] mode=indexing
            tunnel: [w556] -> w527 mode=indexing
            n255 = Build Path(base path=w560, name or relative path=w559) -> (appended path=w558:path)
            n256 = Copy(10:w561, 11:w558) -> (0:w557:errorcluster)  [unwired: 3 in, 2 out]
            n257 = Unbundle By Name(w557) -> ("status"=w556:bool)
          }
          n258 = Not(x=w527) -> (.not. x?=w526:bool[])
          n259 = And Array Elements(Boolean array=w526) -> (logical AND=w529:bool)
          n260 = case shown="True" w529 {
            tunnel: w528 -> [_ w553]
            frame False {
            }
            frame True {
              n261 = Path To String(path=w553) -> (string=w552:string)
              n262 = Concatenate Strings("Data successfully copied from " ("prompt (Delete)"), w552, " to PNILabview. Delete from PNIMatlab?" ("prompt (Delete)")) -> (w548:string)
              n263 = Two Button Dialog(message=w548, 2:"Yes" ("T button name (\"OK\")")) -> (T button?=w547:bool)  [unwired: 1 in]
              n264 = case shown="True" w547 {
                tunnel: w553 -> [_ w554]
                frame False {
                }
                frame True {
                  n265 = Delete(path (use dialog)=w554, entire hierarchy (F)=TRUE) -> ()  [unwired: 3 in, 3 out]
                }
              }
            }
          }
        }
        frame True {
          n266 = One Button Dialog(message="Task files not copied to Labview computer!") -> ()  [unwired: 1 in, 1 out]
        }
      }
      n267 = local read "MLClust"() -> (w525:T5)
    }
    frame "Close" {
      w568 = FALSE ("Load")
      n268 = local read "UDPEvnt"() -> (w573:refnum<k16>)
      n269 = UDP Close(connection ID=w573) -> ()  [unwired: 1 in, 2 out]
      n270 = Bundle By Name(cluster=w571, "CtrlButtons"=T7 {"AcqTraining"=FALSE, "ApplyBaseline"=FALSE, "ApplyTraining"=FALSE, "LoadTrainFile"=FALSE, "CAR"=FALSE, "NIPSpikes"=FALSE, "AcqBaseline"=FALSE, "Stop"=FALSE, "ResetTrial"=FALSE, "TrialSphrs"=FALSE, "HideSphrs"=FALSE, "StartTrials"=FALSE, "AutoPop"=FALSE, "ResetVRE"=FALSE, "StopVRE"=FALSE, "AcqCAR"=FALSE, "ConARD"=FALSE, "Empty2"=FALSE, "Empty1"=FALSE}) -> (w570:T4)
      n271 = local read "UDPCont"() -> (w572:refnum<k16>)
      n272 = UDP Close(connection ID=w572) -> ()  [unwired: 1 in, 2 out]
      n273 = Bundle By Name(cluster=w566, "PresetClust.Load"=w568, "Stim"=w568, "PresetClust.Clear"=w568, "PresetClust.Save"=w568, "StimMode"=enum16{"Off", "Manual", "MSMS", "VRE"}."Off") -> (w565:T3)
      n274 = local read "MLClust"() -> (w569:T5)
    }
  }
  "MLClust" <- w7
  "DecodeClustOut" <- w5
  "EncodeClustOut" <- w3
  "CognitiveLoadOut" <- w1
